vi "211104-VNA RP FLAT.vi"() -> ()   [LabVIEW 2021]
uses:
  b7fd31b3-4c8f-4ae8-a038-7c142e2eb182.vi
  <vilib>/Analysis/baseanly.llb/Mean (DBL).vi
  <vilib>/Utility/file.llb/Write Delimited Spreadsheet (DBL).vi
  <vilib>/Comparison/Equal/Equal Functor/Equal Functor.lvclass
  <vilib>/Analysis/NI_AALBase.lvlib
panel:
  in  "RP VNA SETTING":T1={"F start"=200000, "F stop"=2000500, "Sweep size"=1000, "Decimation"=5000, "F_corr"=0, "Ph_OUT1"=0, "Ph_OUT2"=0, "OUT_Lvl1"=32700, "OUT_Lvl2"=32700, "GPIO"=0}
  in  "Amplitude(1V)":dbl=0.3 format="%#_13g"
  out "RP CONNECT":bool
  in  "VOA Calibration cluster":cluster{"PUMP":dbl[], "PROBE":dbl[]}
  out "TRACK DATA REL NO SMOOTHING":dbl[][](array[numeric])
  out "TRACK DATA ABS NO SMOOTHING":dbl[][](array[numeric])
  in  "BTN SAVE TRACK":bool
  in  "BTN STOP TRACK":bool
  out "TRACK REPOSITERY":path
  out "TRACK DATA REL":dbl[][](array[numeric])
  out "TRACK DATA ABS":dbl[][](array[numeric])
  out "Track File List":path[](array[path])
  out "Track Repositery List":path[](array[path])
  out "CHANNEL CHOSEN":i32
  in  "TRACK-STOP":bool
  out "STATUS":string="STOP"
  out "track data":dbl[](array[numeric])=[495490.5081042979, 495481.56129759253, 495478.2328599854, 495479.84884744807, 495476.377462383, 495478.7819904735]
  out "Information tips":string
  in  "PANEL VNA":bool
  in  "PANEL TRACKING":bool
  in  "BTN STOP":bool
  in  "PANEL GENERAL SETTINGS":bool
  in  "PANEL TRACK SETTINGS":bool
  out "MAIN TAB":T2(tab)
  out "ACQ Indicator":bool
  in  "PUMP":dbl(slide)=100.0 min=0.0 max=100.0 step=0.1 scale=0.0..100.0
  in  "PROBE":dbl(slide)=100.0 min=0.0 max=100.0 step=0.1 scale=0.0..100.0
  in  "BTN RESET VNA":bool
  in  "SPAN":dbl=1900.0 format="%#5.1f"
  in  "STOP":dbl=2000.0 format="%#5.1f"
  in  "CENTER":dbl=1050.0 format="%#5.1f"
  in  "BTN SAVE VNA STG TO TRACK":bool
  in  "BTN AF VNA":bool
  out "MAGNITUDE/PHASE":cluster{cluster{dbl, dbl}[]}[](graph)
  in  "CHANNEL CHOICE VNA":T3(radio)
  in  "BTN Center to max":bool
  in  "BTN ZOOM-":bool
  in  "BTN ZOOM+":bool
  in  "START":dbl=200.0 format="%#5.1f"
  out "SPACING":dbl=1900.0 min=0.0 max=100.0 step=0.5 format="%#5.1f"
  in  "Points N°":i32=1000 min=600 max=5000 step=1 format="%#4.4g"
  in  "BTN LOOP VNA":bool
  in  "BTN RUN VNA":bool
  in  "Hide/Show track data channel":bool[](array[boolean])
  in  "BTN AUTOSAVE RAW DATA":bool=TRUE
  in  "COMMENTS":string
  in  "ASSAY NAME":string
  in  "DELAY AFTER SWITCH (s)":i32
  in  "N°POINTS TO DISPLAY":i32=200
  in  "DISPLAY OPTION":u16(ring) items=["Absolute frequency", "Relative frequency (ppm)"]
  in  "DELAY BETWEEN TRIG (s)":i32
  in  "AVERAGE/POINT":dbl=1.0
  out "LIVE TRACK":dbl[][](graph)
  out "CHANNELS IND TRACK":T3(radio)
  in  "BTN RUN TRACK":bool
  in  "TEMPORAL SMOOTHING":i32=15
  in  "BTN NEW TRACK":bool
  in  "BTN PAUSE TRACK":bool
  in  "CHANNELS PARAMETERS":T4(array[cluster])=[{"START 2"=200.0, "STOP 2"=2000.5, "CENTER 2"=1050.0, "SPAN 2"=1800.0, "CHANNEL TRACK ?"=FALSE, "PUMP"=100.0, "PROBE"=100.0, "Points N° 2"=1000, "SPACING 2"=100.0}, {"START 2"=200.0, "STOP 2"=2000.0, "CENTER 2"=1100.0, "SPAN 2"=1800.0, "CHANNEL TRACK ?"=FALSE, "PUMP"=100.0, "PROBE"=100.0, "Points N° 2"=1000, "SPACING 2"=1800.0}, {"START 2"=200.0, "STOP 2"=2000.0, "CENTER 2"=1100.0, "SPAN 2"=1800.0, "CHANNEL TRACK ?"=FALSE, "PUMP"=100.0, "PROBE"=100.0, "Points N° 2"=1000, "SPACING 2"=1800.0}, {"START 2"=200.0, "STOP 2"=2000.0, "CENTER 2"=1100.0, "SPAN 2"=1800.0, "CHANNEL TRACK ?"=FALSE, "PUMP"=100.0, "PROBE"=100.0, "Points N° 2"=1000, "SPACING 2"=1800.0}, {"START 2"=200.0, "STOP 2"=2000.0, "CENTER 2"=1100.0, "SPAN 2"=1800.0, "CHANNEL TRACK ?"=FALSE, "PUMP"=100.0, "PROBE"=100.0, "Points N° 2"=1000, "SPACING 2"=1800.0}, {"START 2"=200.0, "STOP 2"=2000.0, "CENTER 2"=1100.0, "SPAN 2"=1800.0, "CHANNEL TRACK ?"=FALSE, "PUMP"=100.0, "PROBE"=100.0, "Points N° 2"=1000, "SPACING 2"=1800.0}, {"START 2"=200.0, "STOP 2"=2000.0, "CENTER 2"=1100.0, "SPAN 2"=1800.0, "CHANNEL TRACK ?"=FALSE, "PUMP"=100.0, "PROBE"=100.0, "Points N° 2"=1000, "SPACING 2"=1800.0}, {"START 2"=200.0, "STOP 2"=2000.0, "CENTER 2"=1100.0, "SPAN 2"=1800.0, "CHANNEL TRACK ?"=FALSE, "PUMP"=100.0, "PROBE"=100.0, "Points N° 2"=1000, "SPACING 2"=1800.0}, {"START 2"=200.0, "STOP 2"=2000.0, "CENTER 2"=1100.0, "SPAN 2"=1800.0, "CHANNEL TRACK ?"=FALSE, "PUMP"=100.0, "PROBE"=100.0, "Points N° 2"=1000, "SPACING 2"=1800.0}, {"START 2"=200.0, "STOP 2"=2000.0, "CENTER 2"=1100.0, "SPAN 2"=1800.0, "CHANNEL TRACK ?"=FALSE, "PUMP"=100.0, "PROBE"=100.0, "Points N° 2"=1000, "SPACING 2"=1800.0}, {"START 2"=200.0, "STOP 2"=2000.0, "CENTER 2"=1100.0, "SPAN 2"=1800.0, "CHANNEL TRACK ?"=FALSE, "PUMP"=100.0, "PROBE"=100.0, "Points N° 2"=1000, "SPACING 2"=1800.0}, {"START 2"=200.0, "STOP 2"=2000.0, "CENTER 2"=1100.0, "SPAN 2"=1800.0, "CHANNEL TRACK ?"=FALSE, "PUMP"=100.0, "PROBE"=100.0, "Points N° 2"=1000, "SPACING 2"=1800.0}, {"START 2"=200.0, "STOP 2"=2000.0, "CENTER 2"=1100.0, "SPAN 2"=1800.0, "CHANNEL TRACK ?"=FALSE, "PUMP"=100.0, "PROBE"=100.0, "Points N° 2"=1000, "SPACING 2"=1800.0}, {"START 2"=200.0, "STOP 2"=2000.0, "CENTER 2"=1100.0, "SPAN 2"=1800.0, "CHANNEL TRACK ?"=FALSE, "PUMP"=100.0, "PROBE"=100.0, "Points N° 2"=1000, "SPACING 2"=1800.0}, {"START 2"=200.0, "STOP 2"=2000.0, "CENTER 2"=1100.0, "SPAN 2"=1800.0, "CHANNEL TRACK ?"=FALSE, "PUMP"=100.0, "PROBE"=100.0, "Points N° 2"=1000, "SPACING 2"=1800.0}, {"START 2"=200.0, "STOP 2"=2000.0, "CENTER 2"=1100.0, "SPAN 2"=1800.0, "CHANNEL TRACK ?"=FALSE, "PUMP"=100.0, "PROBE"=100.0, "Points N° 2"=1000, "SPACING 2"=1800.0}] {"SPACING 2" min=0.0 max=100.0 step=0.5; "Points N° 2" min=0 max=100 step=1; "PROBE" min=0.0 max=100.0 step=0.5; "PUMP" min=0.0 max=100.0 step=0.5}
  out "CHANNEL IND SETTINGS":T5(radio)
  in  "TRACK DATA PARAMETERS":cluster{"MAIN FOLDER":path}={"MAIN FOLDER"=path "C:/SensWay Data"}
  in  "SPECTRUM POST PROCESSING PARAMETERS":cluster{"N° SMOOTHING POINTS":i32}={"N° SMOOTHING POINTS"=50}
  in  "AUTOFOCUS PARAMETERS":cluster{"ITERATIONS":i32}={"ITERATIONS"=5}
  in  "CHANNELS":T6
  in  "NETWORK PARAMETERS":cluster{"RP-IP 1":string, "RP-IP 2":string}={"RP-IP 1"="192.168.0.3", "RP-IP 2"="192.168.0.4"}
  in  "VNA DATA CLUSTER":T7
  in  "TRACK DATA CLUSTER":cluster{"CHANNEL":dbl, "KPI 1 TRACK":ext[]}
  out "LOOP ACT":bool
  out "RAW Freq table":dbl[](array[numeric])=[200000.0, 201802.3023023023, 203604.6046046046, 205406.9069069069, 207209.20920920922, 209011.51151151152, 210813.81381381382, 212616.1161161161, 214418.4184184184, 216220.7207207207, 218023.02302302304, 219825.32532532534, 221627.62762762763, 223429.92992992993, 225232.23223223223, 227034.53453453453, 228836.83683683682, 230639.13913913915, 232441.44144144145, 234243.74374374375, 236046.04604604605, 237848.34834834834, 239650.65065065064, 241452.95295295294, 243255.25525525527, 245057.55755755756, 246859.85985985986, 248662.16216216216, 250464.46446446446, 252266.76676676676, 254069.06906906905, 255871.37137137138, 257673.67367367368, 259475.97597597598, 261278.27827827827, 263080.5805805806, 264882.8828828829, 266685.18518518517, 268487.4874874875, 270289.7897897898, 272092.0920920921, 273894.39439439436, 275696.6966966967, 277498.998998999, 279301.3013013013, 281103.6036036036, 282905.9059059059, 284708.2082082082, 286510.51051051053, 288312.8128128128, 290115.1151151151, 291917.4174174174, 293719.7197197197, 295522.02202202205, 297324.3243243243, 299126.6266266266, 300928.9289289289, 302731.23123123124, 304533.5335335335, 306335.83583583584, 308138.1381381381, 309940.44044044043, 311742.74274274276, 313545.04504504503, 315347.34734734736, 317149.6496496496, 318951.95195195195, 320754.2542542543, 322556.55655655655, 324358.8588588588, 326161.16116116114, 327963.4634634635, 329765.76576576574, 331568.06806806807, 333370.37037037034, 335172.67267267266, 336974.974974975, 338777.27727727726, 340579.5795795796, 342381.88188188185, 344184.1841841842, 345986.4864864865, 347788.7887887888, 349591.09109109105, 351393.3933933934, 353195.6956956957, 354997.997997998, 356800.3003003003, 358602.60260260256, 360404.9049049049, 362207.2072072072, 364009.50950950955, 365811.8118118118, 367614.1141141141, 369416.4164164164, 371218.71871871874, 373021.021021021, 374823.3233233233, 376625.6256256256, 378427.9279279279, 380230.23023023026, 382032.5325325325, 383834.8348348348, 385637.1371371371, 387439.43943943945, 389241.7417417418, 391044.04404404404, 392846.3463463463, 394648.64864864864, 396450.95095095097, 398253.25325325324, 400055.5555555555, 401857.85785785783, 403660.16016016016, 405462.4624624625, 407264.76476476475, 409067.067067067, 410869.36936936935, 412671.6716716717, 414473.973973974, 416276.2762762763, 418078.57857857854, 419880.88088088087, 421683.1831831832, 423485.48548548546, 425287.7877877878, 427090.09009009006, 428892.3923923924, 430694.6946946947, 432496.996996997, 434299.29929929925, 436101.6016016016, 437903.9039039039, 439706.20620620623, 441508.5085085085, 443310.81081081077, 445113.1131131131, 446915.4154154154, 448717.7177177177, 450520.02002002, 452322.3223223223, 454124.6246246246, 455926.92692692694, 457729.2292292292, 459531.5315315315, 461333.8338338338, 463136.13613613613, 464938.4384384384, 466740.74074074073, 468543.04304304306, 470345.3453453453, 472147.64764764765, 473949.9499499499, 475752.25225225225, 477554.5545545545, 479356.85685685684, 481159.1591591592, 482961.46146146144, 484763.76376376377, 486566.06606606604, 488368.36836836836, 490170.67067067063, 491972.97297297296, 493775.2752752753, 495577.57757757755, 497379.8798798799, 499182.18218218215, 500984.4844844845, 502786.78678678675, 504589.0890890891, 506391.3913913914, 508193.69369369367, 509995.995995996, 511798.29829829826, 513600.6006006006, 515402.90290290286, 517205.2052052052, 519007.5075075075, 520809.8098098098, 522612.1121121121, 524414.4144144144, 526216.7167167168, 528019.0190190191, 529821.3213213213, 531623.6236236236, 533425.9259259258, 535228.2282282282, 537030.5305305305, 538832.8328328328, 540635.1351351351, 542437.4374374375, 544239.7397397398, 546042.042042042, 547844.3443443443, 549646.6466466465, 551448.9489489489, 553251.2512512512, 555053.5535535535, 556855.8558558559, 558658.1581581582, 560460.4604604605, 562262.7627627627, 564065.065065065, 565867.3673673674, 567669.6696696696, 569471.9719719719, 571274.2742742742, 573076.5765765766, 574878.8788788789, 576681.1811811812, 578483.4834834835, 580285.7857857858, 582088.0880880881, 583890.3903903903, 585692.6926926926, 587494.994994995, 589297.2972972973, 591099.5995995996, 592901.9019019019, 594704.2042042043, 596506.5065065065, 598308.8088088088, 600111.111111111, 601913.4134134133, 603715.7157157157, 605518.018018018, 607320.3203203203, 609122.6226226226, 610924.924924925, 612727.2272272272, 614529.5295295295, 616331.8318318318, 618134.134134134, 619936.4364364364, 621738.7387387387, 623541.041041041, 625343.3433433434, 627145.6456456457, 628947.947947948, 630750.2502502502, 632552.5525525525, 634354.8548548548, 636157.1571571571, 637959.4594594594, 639761.7617617617, 641564.0640640641, 643366.3663663664, 645168.6686686687, 646970.9709709709, 648773.2732732733, 650575.5755755756, 652377.8778778778, 654180.1801801801, 655982.4824824824, 657784.7847847848, 659587.0870870871, 661389.3893893894, 663191.6916916918, 664993.993993994, 666796.2962962963, 668598.5985985985, 670400.9009009008, 672203.2032032032, 674005.5055055055, 675807.8078078078, 677610.1101101101, 679412.4124124125, 681214.7147147147, 683017.017017017, 684819.3193193192, 686621.6216216215, 688423.9239239239, 690226.2262262262, 692028.5285285285, 693830.8308308308, 695633.1331331332, 697435.4354354354, 699237.7377377377, 701040.04004004, 702842.3423423423, 704644.6446446446, 706446.9469469469, 708249.2492492492, 710051.5515515516, 711853.8538538539, 713656.1561561562, 715458.4584584584, 717260.7607607607, 719063.063063063, 720865.3653653653, 722667.6676676676, 724469.9699699699, 726272.2722722723, 728074.5745745746, 729876.8768768768, 731679.1791791791, 733481.4814814815, 735283.7837837838, 737086.0860860861, 738888.3883883883, 740690.6906906907, 742492.992992993, 744295.2952952953, 746097.5975975975, 747899.8998998998, 749702.2022022022, 751504.5045045045, 753306.8068068068, 755109.109109109, 756911.4114114114, 758713.7137137137, 760516.016016016, 762318.3183183183, 764120.6206206206, 765922.9229229229, 767725.2252252252, 769527.5275275275, 771329.8298298299, 773132.1321321321, 774934.4344344344, 776736.7367367367, 778539.039039039, 780341.3413413413, 782143.6436436436, 783945.9459459459, 785748.2482482482, 787550.5505505506, 789352.8528528528, 791155.1551551551, 792957.4574574574, 794759.7597597598, 796562.0620620621, 798364.3643643643, 800166.6666666666, 801968.968968969, 803771.2712712713, 805573.5735735735, 807375.8758758758, 809178.1781781781, 810980.4804804805, 812782.7827827828, 814585.085085085, 816387.3873873873, 818189.6896896897, 819991.991991992, 821794.2942942943, 823596.5965965965, 825398.8988988989, 827201.2012012012, 829003.5035035035, 830805.8058058057, 832608.108108108, 834410.4104104104, 836212.7127127127, 838015.015015015, 839817.3173173172, 841619.6196196196, 843421.9219219219, 845224.2242242242, 847026.5265265265, 848828.8288288288, 850631.1311311311, 852433.4334334334, 854235.7357357357, 856038.0380380381, 857840.3403403403, 859642.6426426426, 861444.9449449449, 863247.2472472473, 865049.5495495495, 866851.8518518518, 868654.1541541541, 870456.4564564564, 872258.7587587588, 874061.061061061, 875863.3633633633, 877665.6656656656, 879467.967967968, 881270.2702702703, 883072.5725725725, 884874.8748748748, 886677.1771771772, 888479.4794794795, 890281.7817817817, 892084.084084084, 893886.3863863864, 895688.6886886887, 897490.990990991, 899293.2932932932, 901095.5955955955, 902897.8978978979, 904700.2002002002, 906502.5025025025, 908304.8048048047, 910107.1071071071, 911909.4094094094, 913711.7117117117, 915514.0140140139, 917316.3163163163, 919118.6186186186, 920920.9209209209, 922723.2232232232, 924525.5255255254, 926327.8278278278, 928130.1301301301, 929932.4324324324, 931734.7347347348, 933537.037037037, 935339.3393393393, 937141.6416416416, 938943.943943944, 940746.2462462463, 942548.5485485485, 944350.8508508508, 946153.1531531531, 947955.4554554555, 949757.7577577577, 951560.06006006, 953362.3623623623, 955164.6646646647, 956966.966966967, 958769.2692692692, 960571.5715715715, 962373.8738738738, 964176.1761761762, 965978.4784784785, 967780.7807807807, 969583.083083083, 971385.3853853854, 973187.6876876877, 974989.9899899899, 976792.2922922922, 978594.5945945946, 980396.8968968969, 982199.1991991992, 984001.5015015014, 985803.8038038037, 987606.1061061061, 989408.4084084084, 991210.7107107107, 993013.0130130129, 994815.3153153153, 996617.6176176176, 998419.9199199199, 1000222.2222222221, 1002024.5245245245, 1003826.8268268268, 1005629.1291291291, 1007431.4314314314, 1009233.7337337337, 1011036.036036036, 1012838.3383383383, 1014640.6406406406, 1016442.942942943, 1018245.2452452452, 1020047.5475475475, 1021849.8498498498, 1023652.1521521521, 1025454.4544544544, 1027256.7567567567, 1029059.059059059, 1030861.3613613613, 1032663.6636636637, 1034465.9659659659, 1036268.2682682682, 1038070.5705705705, 1039872.8728728729, 1041675.1751751752, 1043477.4774774774, 1045279.7797797797, 1047082.082082082, 1048884.3843843844, 1050686.6866866867, 1052488.988988989, 1054291.2912912914, 1056093.5935935937, 1057895.895895896, 1059698.198198198, 1061500.5005005004, 1063302.8028028028, 1065105.105105105, 1066907.4074074074, 1068709.7097097095, 1070512.0120120118, 1072314.3143143142, 1074116.6166166165, 1075918.9189189188, 1077721.2212212211, 1079523.5235235235, 1081325.8258258258, 1083128.1281281281, 1084930.4304304305, 1086732.7327327328, 1088535.035035035, 1090337.3373373374, 1092139.6396396398, 1093941.9419419419, 1095744.2442442442, 1097546.5465465465, 1099348.8488488488, 1101151.1511511512, 1102953.4534534533, 1104755.7557557556, 1106558.058058058, 1108360.3603603602, 1110162.6626626626, 1111964.964964965, 1113767.2672672672, 1115569.5695695695, 1117371.8718718719, 1119174.1741741742, 1120976.4764764765, 1122778.7787787789, 1124581.0810810812, 1126383.3833833835, 1128185.6856856856, 1129987.987987988, 1131790.2902902903, 1133592.5925925926, 1135394.894894895, 1137197.197197197, 1138999.4994994993, 1140801.8018018017, 1142604.104104104, 1144406.4064064063, 1146208.7087087086, 1148011.011011011, 1149813.3133133133, 1151615.6156156156, 1153417.917917918, 1155220.2202202203, 1157022.5225225226, 1158824.824824825, 1160627.1271271273, 1162429.4294294294, 1164231.7317317317, 1166034.034034034, 1167836.3363363363, 1169638.6386386384, 1171440.9409409408, 1173243.243243243, 1175045.5455455454, 1176847.8478478477, 1178650.15015015, 1180452.4524524524, 1182254.7547547547, 1184057.057057057, 1185859.3593593594, 1187661.6616616617, 1189463.963963964, 1191266.2662662663, 1193068.5685685687, 1194870.8708708708, 1196673.173173173, 1198475.4754754754, 1200277.7777777778, 1202080.08008008, 1203882.3823823822, 1205684.6846846845, 1207486.9869869868, 1209289.2892892892, 1211091.5915915915, 1212893.8938938938, 1214696.1961961961, 1216498.4984984985, 1218300.8008008008, 1220103.103103103, 1221905.4054054054, 1223707.7077077078, 1225510.01001001, 1227312.3123123124, 1229114.6146146145, 1230916.9169169168, 1232719.2192192192, 1234521.5215215215, 1236323.8238238238, 1238126.126126126, 1239928.4284284282, 1241730.7307307306, 1243533.033033033, 1245335.3353353352, 1247137.6376376376, 1248939.9399399399, 1250742.2422422422, 1252544.5445445445, 1254346.8468468469, 1256149.1491491492, 1257951.4514514515, 1259753.7537537536, 1261556.056056056, 1263358.3583583583, 1265160.6606606606, 1266962.962962963, 1268765.2652652652, 1270567.5675675676, 1272369.86986987, 1274172.1721721722, 1275974.4744744743, 1277776.7767767766, 1279579.079079079, 1281381.3813813813, 1283183.6836836836, 1284985.985985986, 1286788.2882882883, 1288590.5905905906, 1290392.892892893, 1292195.195195195, 1293997.4974974974, 1295799.7997997997, 1297602.102102102, 1299404.4044044043, 1301206.7067067067, 1303009.009009009, 1304811.3113113113, 1306613.6136136136, 1308415.915915916, 1310218.218218218, 1312020.5205205204, 1313822.8228228227, 1315625.125125125, 1317427.4274274274, 1319229.7297297297, 1321032.032032032, 1322834.3343343344, 1324636.6366366367, 1326438.9389389388, 1328241.241241241, 1330043.5435435434, 1331845.8458458458, 1333648.148148148, 1335450.4504504504, 1337252.7527527527, 1339055.055055055, 1340857.3573573574, 1342659.6596596597, 1344461.9619619618, 1346264.2642642641, 1348066.5665665665, 1349868.8688688688, 1351671.1711711711, 1353473.4734734735, 1355275.7757757758, 1357078.078078078, 1358880.3803803804, 1360682.6826826825, 1362484.9849849849, 1364287.2872872872, 1366089.5895895895, 1367891.8918918918, 1369694.1941941942, 1371496.4964964965, 1373298.7987987988, 1375101.1011011011, 1376903.4034034032, 1378705.7057057056, 1380508.008008008, 1382310.3103103102, 1384112.6126126125, 1385914.9149149149, 1387717.2172172172, 1389519.5195195195, 1391321.8218218219, 1393124.1241241242, 1394926.4264264263, 1396728.7287287286, 1398531.031031031, 1400333.3333333333, 1402135.6356356356, 1403937.937937938, 1405740.2402402402, 1407542.5425425426, 1409344.844844845, 1411147.147147147, 1412949.4494494493, 1414751.7517517516, 1416554.054054054, 1418356.3563563563, 1420158.6586586586, 1421960.960960961, 1423763.2632632633, 1425565.5655655656, 1427367.867867868, 1429170.17017017, 1430972.4724724723, 1432774.7747747747, 1434577.077077077, 1436379.3793793793, 1438181.6816816817, 1439983.983983984, 1441786.2862862863, 1443588.5885885886, 1445390.8908908907, 1447193.193193193, 1448995.4954954954, 1450797.7977977977, 1452600.1001001, 1454402.4024024024, 1456204.7047047047, 1458007.007007007, 1459809.3093093093, 1461611.6116116114, 1463413.9139139138, 1465216.216216216, 1467018.5185185184, 1468820.8208208208, 1470623.123123123, 1472425.4254254254, 1474227.7277277277, 1476030.03003003, 1477832.3323323324, 1479634.6346346345, 1481436.9369369368, 1483239.2392392391, 1485041.5415415415, 1486843.8438438438, 1488646.146146146, 1490448.4484484484, 1492250.7507507508, 1494053.053053053, 1495855.3553553552, 1497657.6576576575, 1499459.9599599598, 1501262.2622622622, 1503064.5645645645, 1504866.8668668668, 1506669.1691691692, 1508471.4714714715, 1510273.7737737738, 1512076.0760760761, 1513878.3783783782, 1515680.6806806806, 1517482.9829829829, 1519285.2852852852, 1521087.5875875875, 1522889.8898898899, 1524692.1921921922, 1526494.4944944945, 1528296.7967967968, 1530099.099099099, 1531901.4014014013, 1533703.7037037036, 1535506.006006006, 1537308.3083083082, 1539110.6106106106, 1540912.912912913, 1542715.2152152152, 1544517.5175175176, 1546319.8198198196, 1548122.122122122, 1549924.4244244243, 1551726.7267267266, 1553529.029029029, 1555331.3313313313, 1557133.6336336336, 1558935.935935936, 1560738.2382382383, 1562540.5405405406, 1564342.8428428427, 1566145.145145145, 1567947.4474474473, 1569749.7497497497, 1571552.052052052, 1573354.3543543543, 1575156.6566566566, 1576958.958958959, 1578761.2612612613, 1580563.5635635634, 1582365.8658658657, 1584168.168168168, 1585970.4704704704, 1587772.7727727727, 1589575.075075075, 1591377.3773773774, 1593179.6796796797, 1594981.981981982, 1596784.2842842843, 1598586.5865865864, 1600388.8888888888, 1602191.191191191, 1603993.4934934934, 1605795.7957957957, 1607598.098098098, 1609400.4004004004, 1611202.7027027027, 1613005.005005005, 1614807.3073073071, 1616609.6096096095, 1618411.9119119118, 1620214.2142142141, 1622016.5165165165, 1623818.8188188188, 1625621.121121121, 1627423.4234234234, 1629225.7257257258, 1631028.0280280279, 1632830.3303303302, 1634632.6326326325, 1636434.9349349348, 1638237.2372372372, 1640039.5395395395, 1641841.8418418418, 1643644.1441441441, 1645446.4464464465, 1647248.7487487488, 1649051.051051051, 1650853.3533533532, 1652655.6556556555, 1654457.9579579579, 1656260.2602602602, 1658062.5625625625, 1659864.8648648649, 1661667.1671671672, 1663469.4694694695, 1665271.7717717716, 1667074.074074074, 1668876.3763763763, 1670678.6786786786, 1672480.980980981, 1674283.2832832832, 1676085.5855855856, 1677887.887887888, 1679690.1901901902, 1681492.4924924925, 1683294.7947947946, 1685097.097097097, 1686899.3993993993, 1688701.7017017016, 1690504.004004004, 1692306.3063063063, 1694108.6086086086, 1695910.910910911, 1697713.2132132133, 1699515.5155155153, 1701317.8178178177, 1703120.12012012, 1704922.4224224223, 1706724.7247247247, 1708527.027027027, 1710329.3293293293, 1712131.6316316316, 1713933.933933934, 1715736.236236236, 1717538.5385385384, 1719340.8408408407, 1721143.143143143, 1722945.4454454454, 1724747.7477477477, 1726550.05005005, 1728352.3523523523, 1730154.6546546547, 1731956.956956957, 1733759.259259259, 1735561.5615615614, 1737363.8638638637, 1739166.166166166, 1740968.4684684684, 1742770.7707707707, 1744573.073073073, 1746375.3753753754, 1748177.6776776777, 1749979.9799799798, 1751782.2822822821, 1753584.5845845845, 1755386.8868868868, 1757189.189189189, 1758991.4914914914, 1760793.7937937938, 1762596.096096096, 1764398.3983983984, 1766200.7007007005, 1768003.0030030028, 1769805.3053053052, 1771607.6076076075, 1773409.9099099098, 1775212.2122122122, 1777014.5145145145, 1778816.8168168168, 1780619.1191191191, 1782421.4214214215, 1784223.7237237236, 1786026.0260260259, 1787828.3283283282, 1789630.6306306305, 1791432.9329329329, 1793235.2352352352, 1795037.5375375375, 1796839.8398398398, 1798642.1421421422, 1800444.4444444443, 1802246.7467467466, 1804049.049049049, 1805851.3513513512, 1807653.6536536536, 1809455.955955956, 1811258.2582582582, 1813060.5605605606, 1814862.8628628629, 1816665.1651651652, 1818467.4674674673, 1820269.7697697696, 1822072.072072072, 1823874.3743743743, 1825676.6766766766, 1827478.978978979, 1829281.2812812813, 1831083.5835835836, 1832885.885885886, 1834688.188188188, 1836490.4904904903, 1838292.7927927927, 1840095.095095095, 1841897.3973973973, 1843699.6996996996, 1845502.002002002, 1847304.3043043043, 1849106.6066066066, 1850908.9089089087, 1852711.211211211, 1854513.5135135134, 1856315.8158158157, 1858118.118118118, 1859920.4204204204, 1861722.7227227227, 1863525.025025025, 1865327.3273273273, 1867129.6296296297, 1868931.9319319318, 1870734.234234234, 1872536.5365365364, 1874338.8388388387, 1876141.141141141, 1877943.4434434434, 1879745.7457457457, 1881548.048048048, 1883350.3503503504, 1885152.6526526525, 1886954.9549549548, 1888757.2572572571, 1890559.5595595594, 1892361.8618618618, 1894164.164164164, 1895966.4664664664, 1897768.7687687688, 1899571.071071071, 1901373.3733733734, 1903175.6756756755, 1904977.9779779778, 1906780.2802802802, 1908582.5825825825, 1910384.8848848848, 1912187.1871871871, 1913989.4894894895, 1915791.7917917918, 1917594.0940940941, 1919396.3963963962, 1921198.6986986985, 1923001.0010010009, 1924803.3033033032, 1926605.6056056055, 1928407.9079079079, 1930210.2102102102, 1932012.5125125125, 1933814.8148148148, 1935617.117117117, 1937419.4194194193, 1939221.7217217216, 1941024.024024024, 1942826.3263263262, 1944628.6286286286, 1946430.930930931, 1948233.2332332332, 1950035.5355355355, 1951837.8378378379, 1953640.14014014, 1955442.4424424423, 1957244.7447447446, 1959047.047047047, 1960849.3493493493, 1962651.6516516516, 1964453.953953954, 1966256.2562562563, 1968058.5585585586, 1969860.8608608607, 1971663.163163163, 1973465.4654654653, 1975267.7677677677, 1977070.07007007, 1978872.3723723723, 1980674.6746746746, 1982476.976976977, 1984279.2792792793, 1986081.5815815816, 1987883.8838838837, 1989686.186186186, 1991488.4884884884, 1993290.7907907907, 1995093.093093093, 1996895.3953953953, 1998697.6976976977, 2000500.0]
  in  "ENABLE INTERNAL MODULATION":bool=TRUE
  in  "VNA DATA CLUSTER TBL":T8(array[cluster])=[{"CHANNEL"=0.0, "FREQUENCY TABLE"=[0.0], "MAGNITUDE TABLE"=[0.0], "PHASE TABLE"=[0.0]}, {"CHANNEL"=1.0, "FREQUENCY TABLE"=[], "MAGNITUDE TABLE"=[], "PHASE TABLE"=[]}, {"CHANNEL"=2.0, "FREQUENCY TABLE"=[], "MAGNITUDE TABLE"=[], "PHASE TABLE"=[]}, {"CHANNEL"=3.0, "FREQUENCY TABLE"=[], "MAGNITUDE TABLE"=[], "PHASE TABLE"=[]}, {"CHANNEL"=4.0, "FREQUENCY TABLE"=[], "MAGNITUDE TABLE"=[], "PHASE TABLE"=[]}, {"CHANNEL"=5.0, "FREQUENCY TABLE"=[], "MAGNITUDE TABLE"=[], "PHASE TABLE"=[]}, {"CHANNEL"=6.0, "FREQUENCY TABLE"=[], "MAGNITUDE TABLE"=[], "PHASE TABLE"=[]}, {"CHANNEL"=7.0, "FREQUENCY TABLE"=[], "MAGNITUDE TABLE"=[], "PHASE TABLE"=[]}, {"CHANNEL"=8.0, "FREQUENCY TABLE"=[], "MAGNITUDE TABLE"=[], "PHASE TABLE"=[]}, {"CHANNEL"=9.0, "FREQUENCY TABLE"=[], "MAGNITUDE TABLE"=[], "PHASE TABLE"=[]}, {"CHANNEL"=10.0, "FREQUENCY TABLE"=[], "MAGNITUDE TABLE"=[], "PHASE TABLE"=[]}, {"CHANNEL"=11.0, "FREQUENCY TABLE"=[], "MAGNITUDE TABLE"=[], "PHASE TABLE"=[]}, {"CHANNEL"=12.0, "FREQUENCY TABLE"=[], "MAGNITUDE TABLE"=[], "PHASE TABLE"=[]}, {"CHANNEL"=13.0, "FREQUENCY TABLE"=[], "MAGNITUDE TABLE"=[], "PHASE TABLE"=[]}, {"CHANNEL"=14.0, "FREQUENCY TABLE"=[], "MAGNITUDE TABLE"=[], "PHASE TABLE"=[]}, {"CHANNEL"=15.0, "FREQUENCY TABLE"=[], "MAGNITUDE TABLE"=[], "PHASE TABLE"=[]}]
  in  "TRACK DATA CLUSTER TBL":cluster{"CHANNEL":dbl, "KPI 1 TRACK":ext[]}[](array[cluster])
  in  "VNA Settings cluster":T9={"START 2"=200.0, "STOP 2"=2000.5, "CENTER 2"=1050.0, "SPAN 2"=1901.0, "CHANNEL TRACK ?"=FALSE, "PUMP"=100.0, "PROBE"=100.0, "Points N° 2"=1000, "SPACING 2"=1901.0} {"SPACING 2" min=0.0 max=100.0 step=0.5; "Points N° 2" min=0 max=100 step=1; "PROBE" min=0.0 max=100.0 step=0.5; "PUMP" min=0.0 max=100.0 step=0.5}
  # "E"
  # "POINTS"
  # "SPACING"
  # "TRACK ?"
  # "START"
  # "STOP"
  # "CENTER"
  # "SPAN"
  # "PROBE"
  # "PUMP"
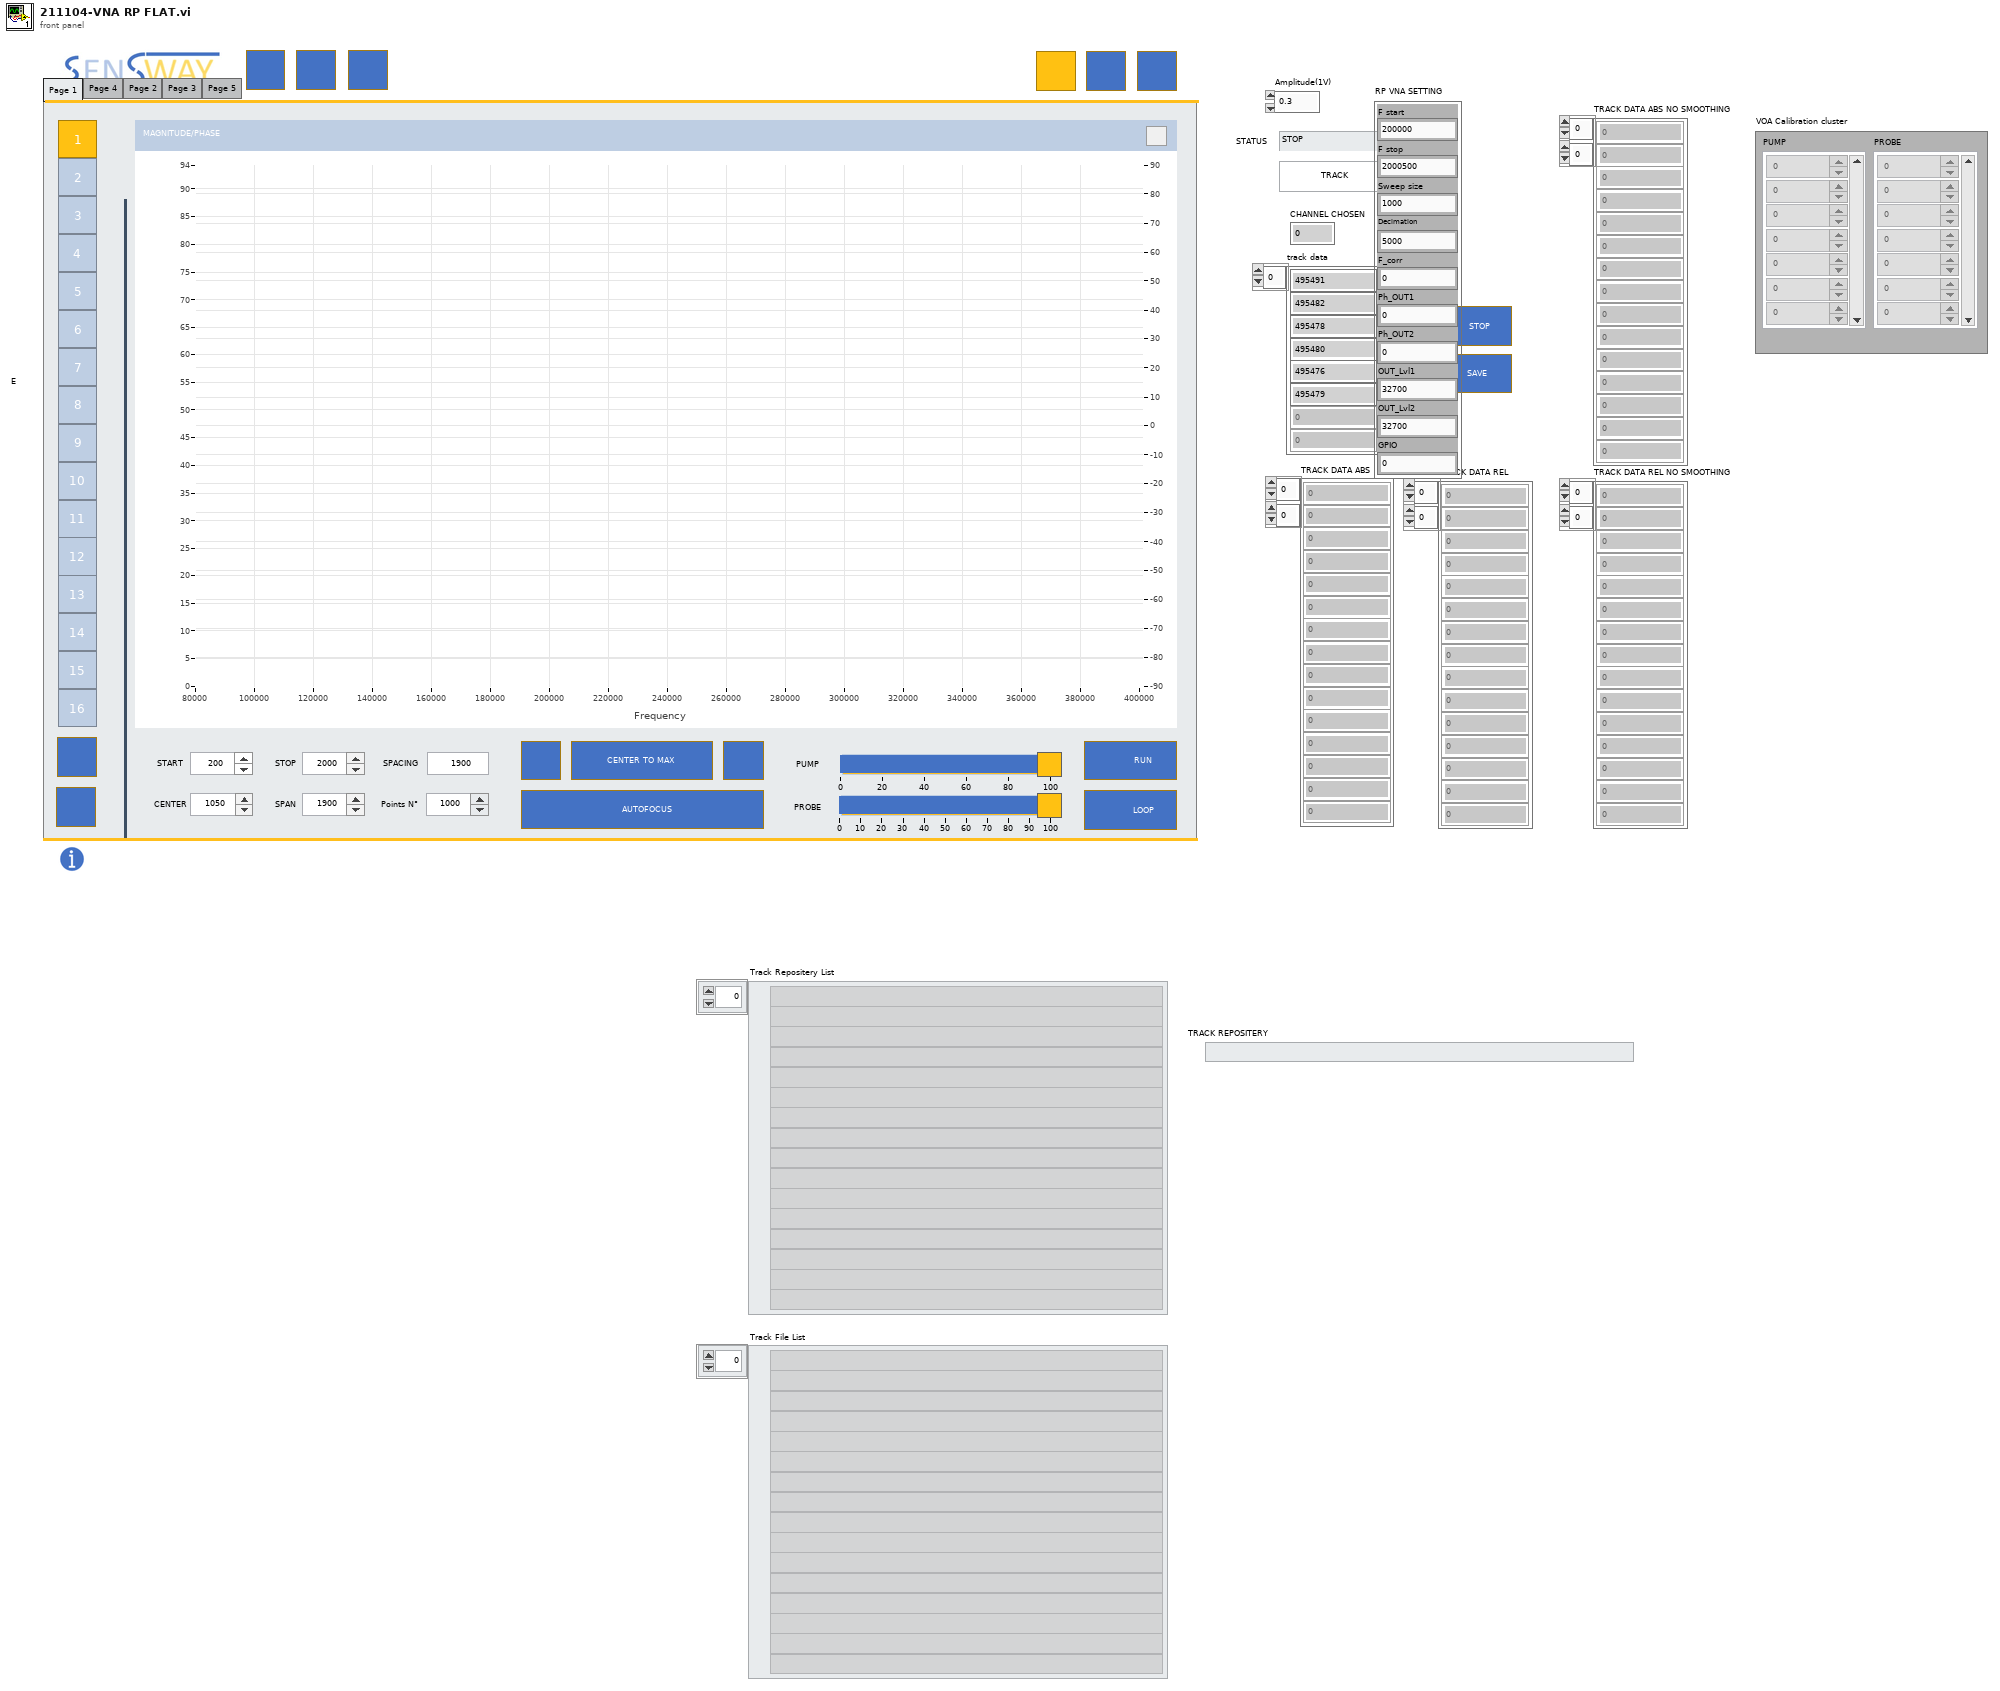
[diagram p1: front panel]
types:
  T1 = cluster{"F start":u32, "F stop":u32, "Sweep size":u32, "Decimation":u32, "F_corr":u32, "Ph_OUT1":u32, "Ph_OUT2":u32, "OUT_Lvl1":u32, "OUT_Lvl2":u32, "GPIO":u32}
  T2 = enum32{"Page 1", "Page 4", "Page 2", "Page 3", "Page 5"}
  T3 = enum32{"Button 1", "Button 2", "Button 3", "Sélection radio 4", "Sélection radio 5", "Sélection radio 6", "Sélection radio 7", "Sélection radio 8", "Sélection radio 9", "Sélection radio 10", "Sélection radio 11", "Sélection radio 12", "Sélection radio 13", "Sélection radio 14", "Sélection radio 15", "Sélection radio 16"}
  T4 = cluster{"START 2":dbl, "STOP 2":dbl, "CENTER 2":dbl, "SPAN 2":dbl, "CHANNEL TRACK ?":bool, "PUMP":dbl, "PROBE":dbl, "Points N° 2":i32, "SPACING 2":dbl}[]
  T5 = enum32{"No Selection", "Button 1", "Button 2", "Button 3", "Sélection radio 4", "Sélection radio 5", "Sélection radio 6", "Sélection radio 7", "Sélection radio 8", "Sélection radio 9", "Sélection radio 10", "Sélection radio 11", "Sélection radio 12", "Sélection radio 13", "Sélection radio 14", "Sélection radio 15", "Sélection radio 16"}
  T6 = cluster{"CHANNEL 1":bool, "CHANNEL 2":bool, "CHANNEL 3":bool, "CHANNEL 4":bool, "CHANNEL 5":bool, "CHANNEL 6":bool, "CHANNEL 7":bool, "CHANNEL 8":bool, "CHANNEL 9":bool, "CHANNEL 10":bool, "CHANNEL 11":bool, "CHANNEL 12":bool, "CHANNEL 13":bool, "CHANNEL 14":bool, "CHANNEL 15":bool, "CHANNEL 16":bool}
  T7 = cluster{"CHANNEL":dbl, "FREQUENCY TABLE":ext[], "MAGNITUDE TABLE":ext[], "PHASE TABLE":ext[]}
  T8 = cluster{"CHANNEL":dbl, "FREQUENCY TABLE":ext[], "MAGNITUDE TABLE":ext[], "PHASE TABLE":ext[]}[]
  T9 = cluster{"START 2":dbl, "STOP 2":dbl, "CENTER 2":dbl, "SPAN 2":dbl, "CHANNEL TRACK ?":bool, "PUMP":dbl, "PROBE":dbl, "Points N° 2":i32, "SPACING 2":dbl}
  T10 = enum16{"Freq start", "Freq stop", "Sweep size", "Decimation rate", "Freq corr", "Phase output 1", "Phase output 2", "Output level 1", "Output level 2", "GPIO", "SWEEP START"}
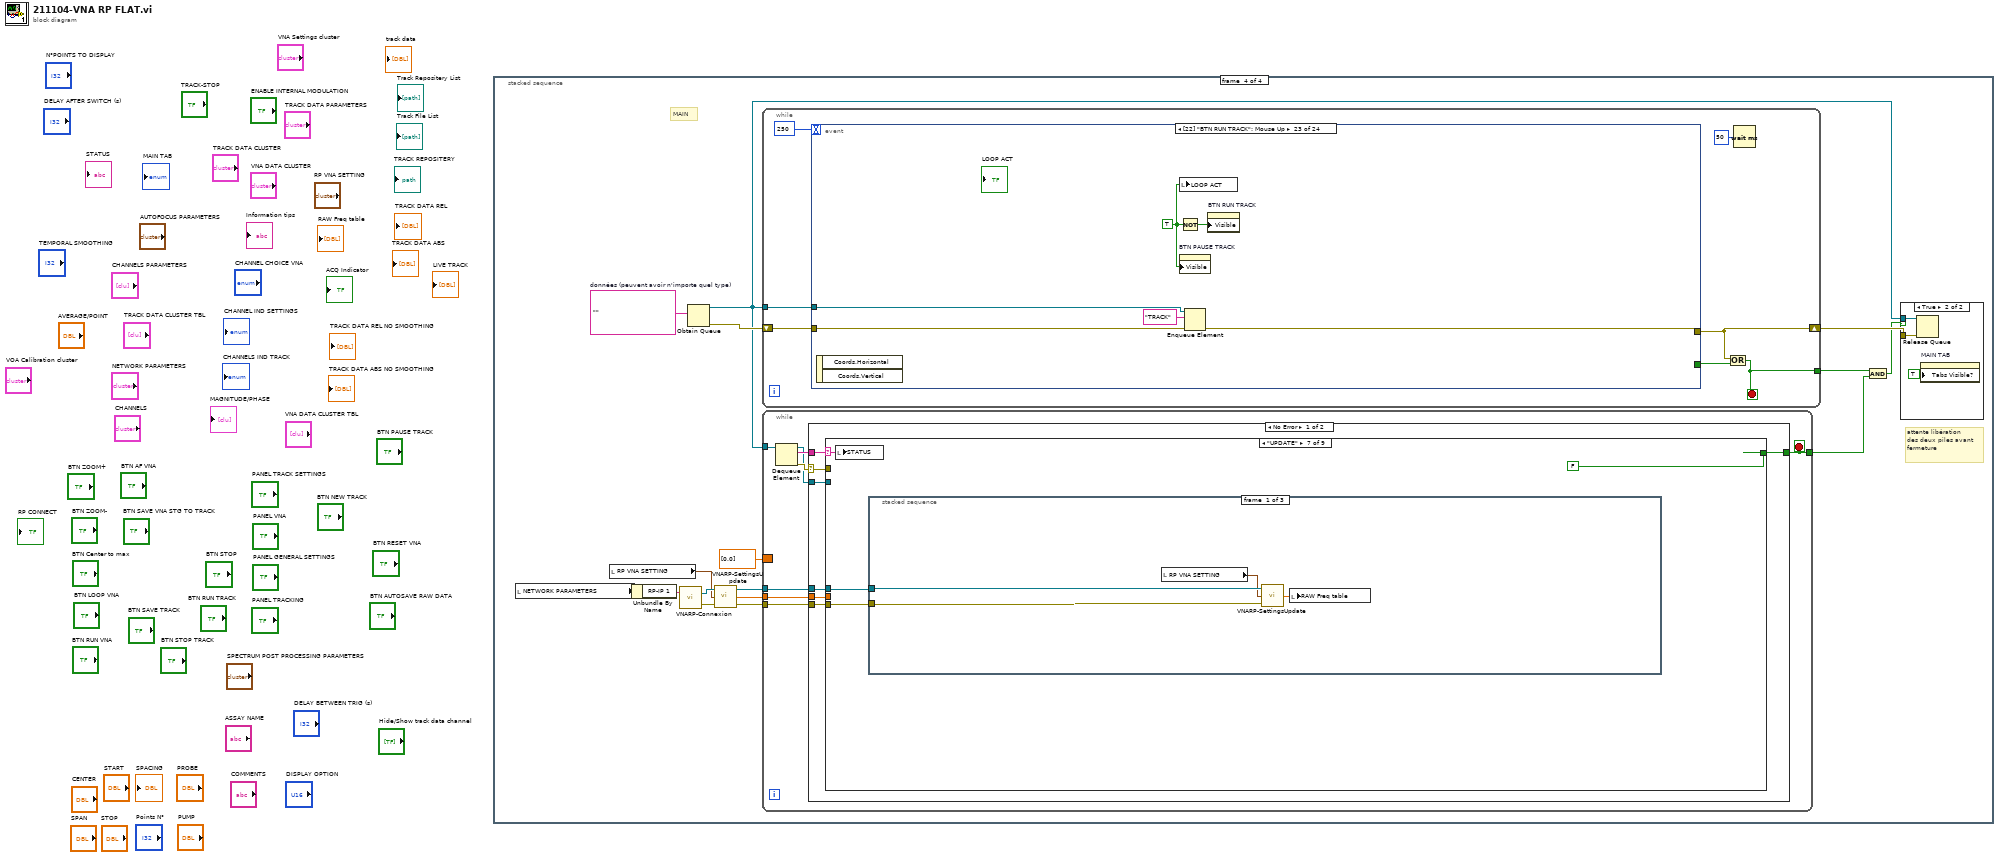
[diagram p0: block diagram]
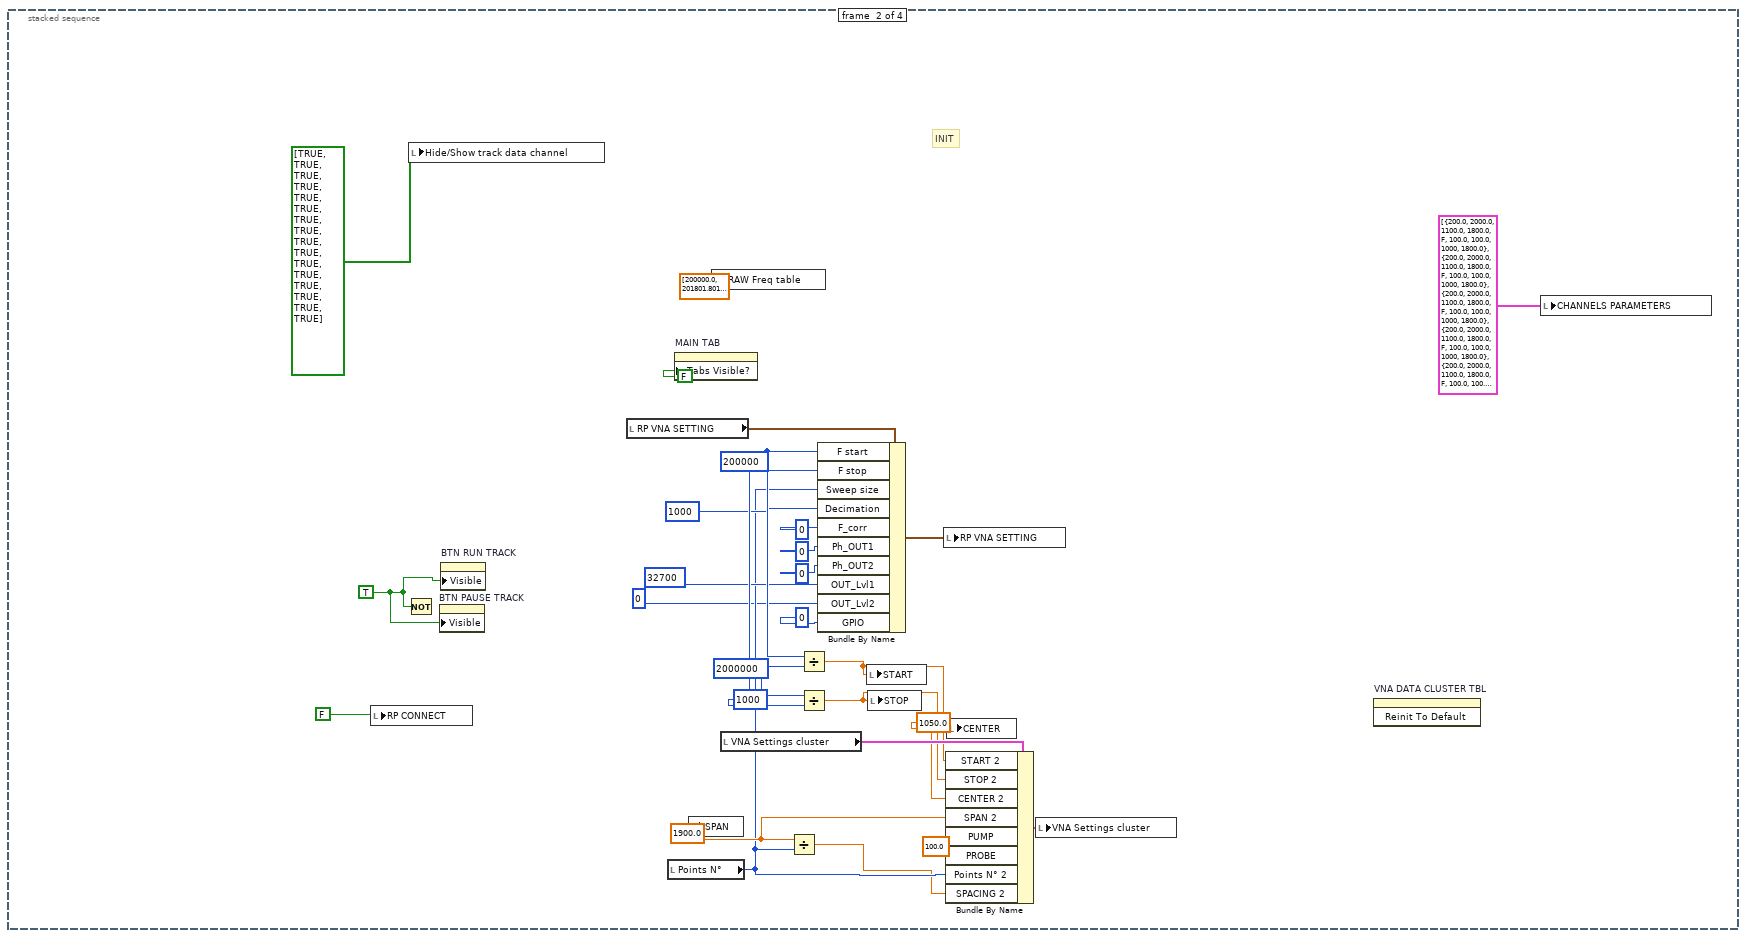
[diagram p3: hidden frame]
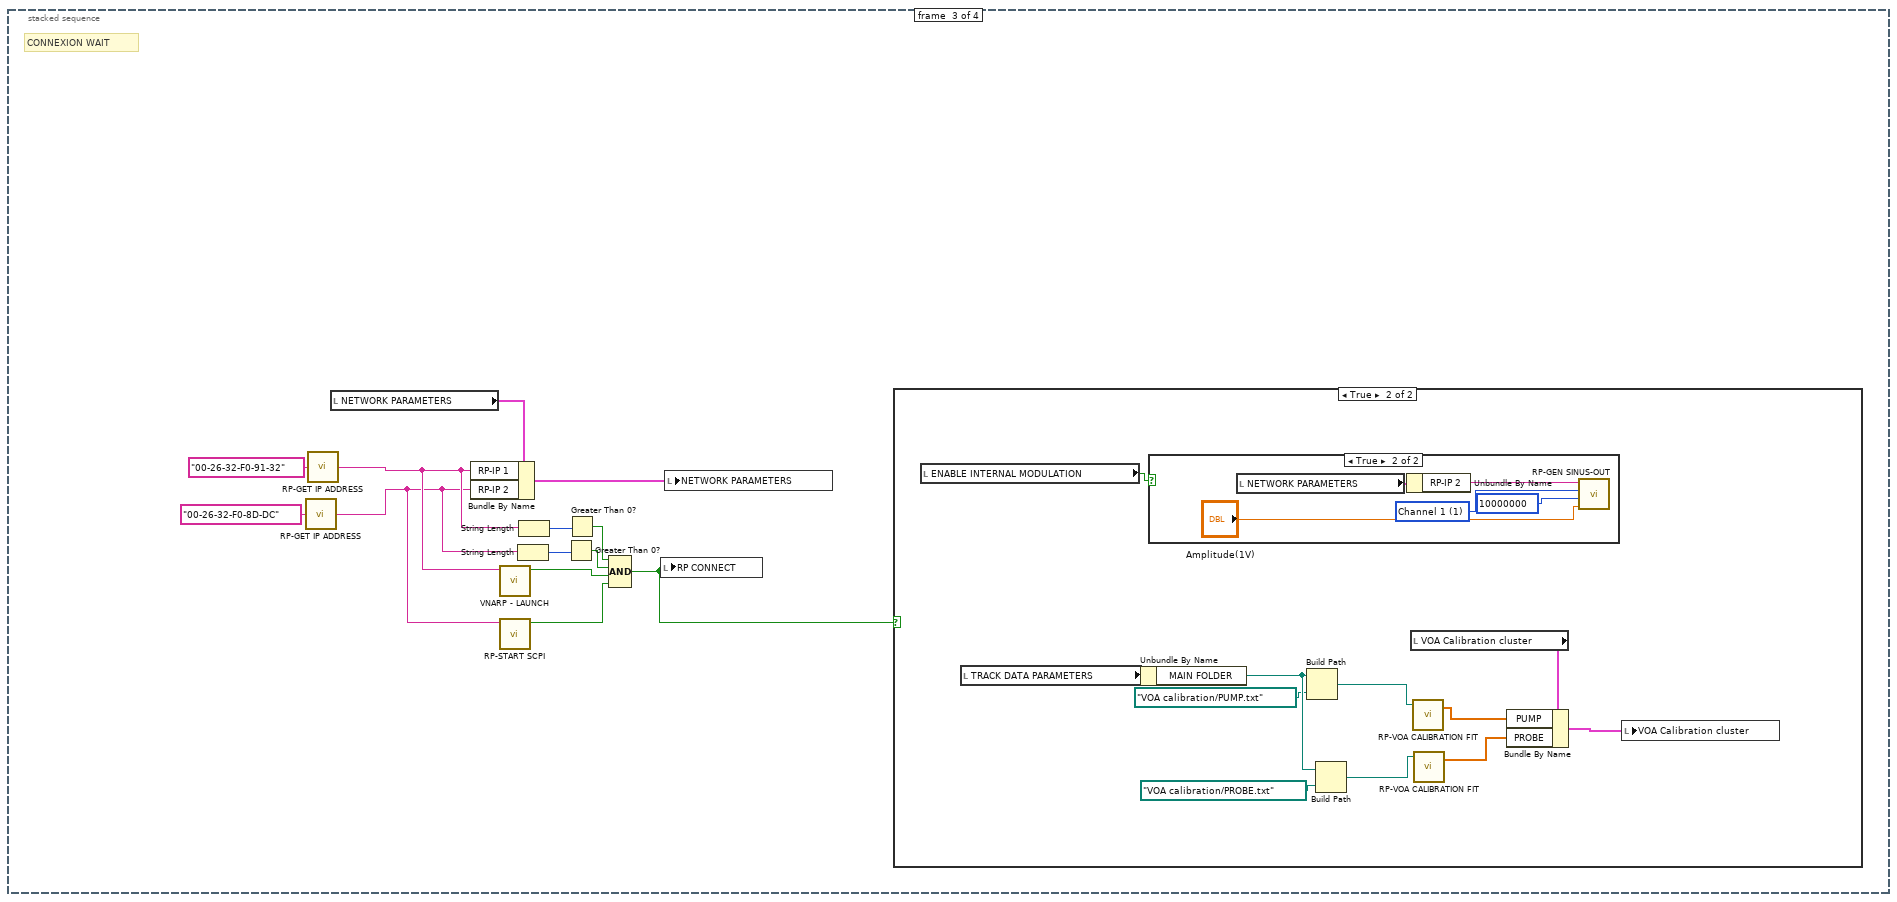
[diagram p4: hidden frame]
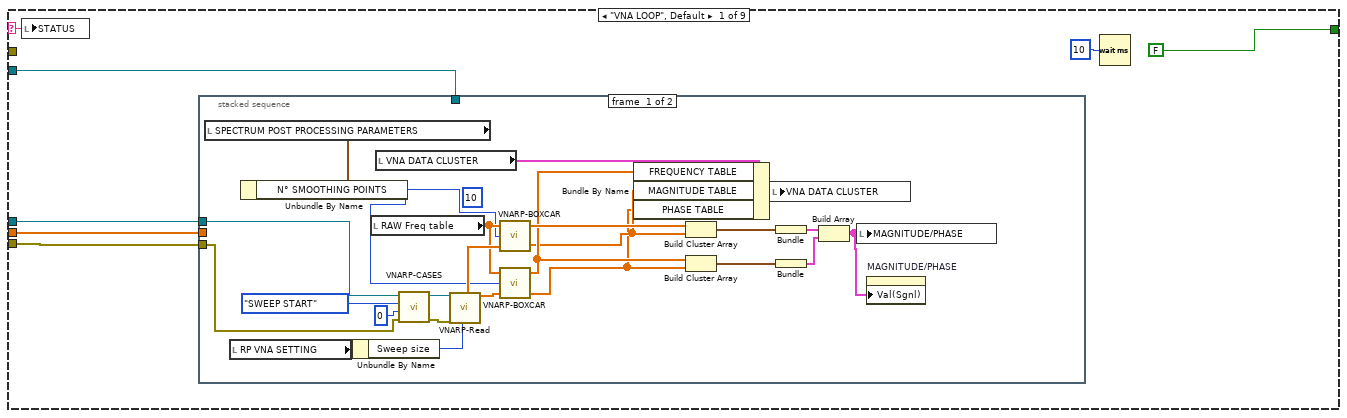
[diagram p8: hidden frame]
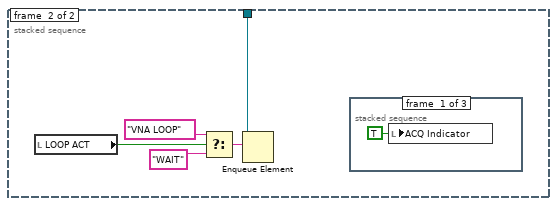
[diagram p9: hidden frame]
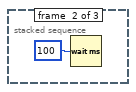
[diagram p10: hidden frame]
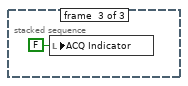
[diagram p11: hidden frame]
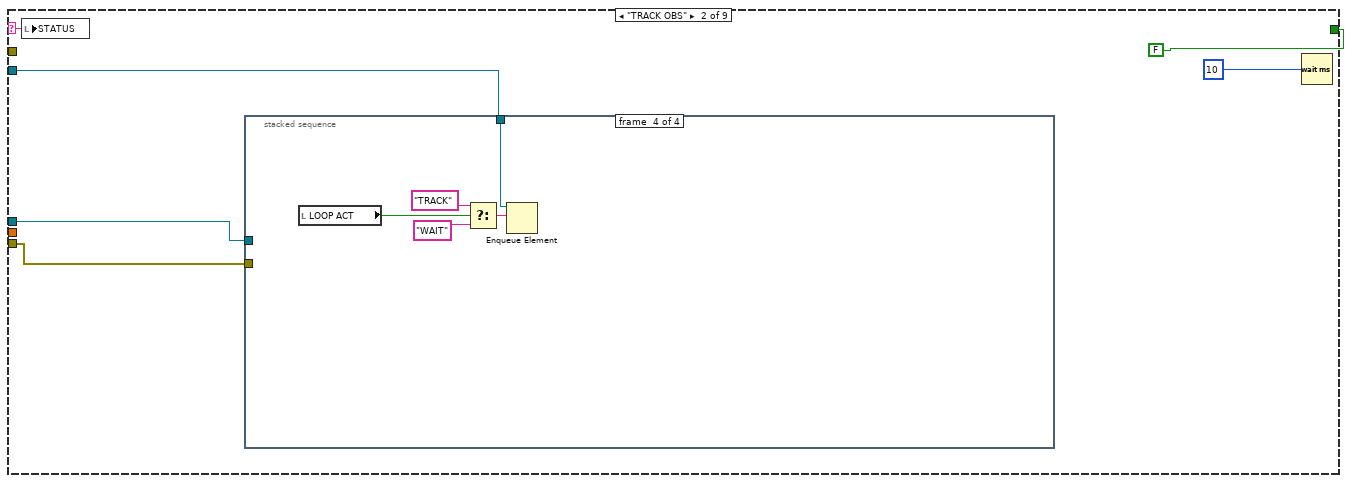
[diagram p12: hidden frame]
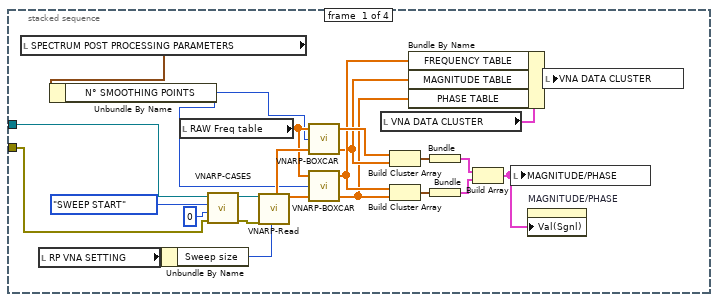
[diagram p13: hidden frame]
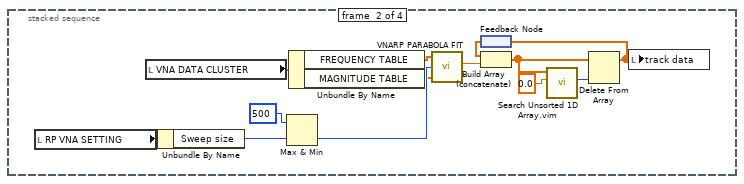
[diagram p14: hidden frame]
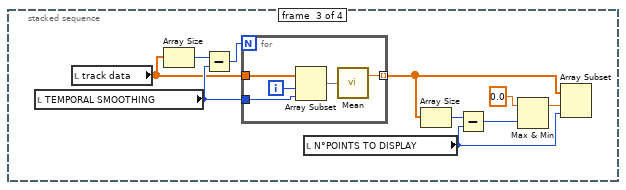
[diagram p15: hidden frame]
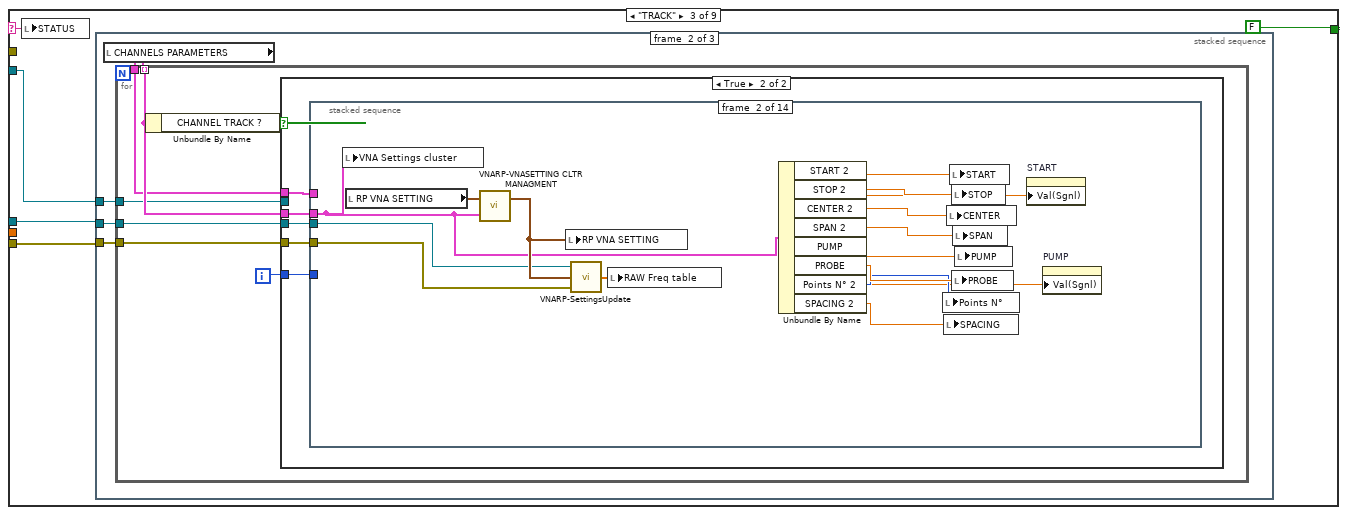
[diagram p16: hidden frame]
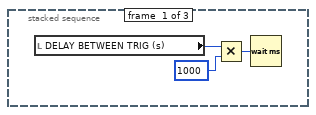
[diagram p17: hidden frame]
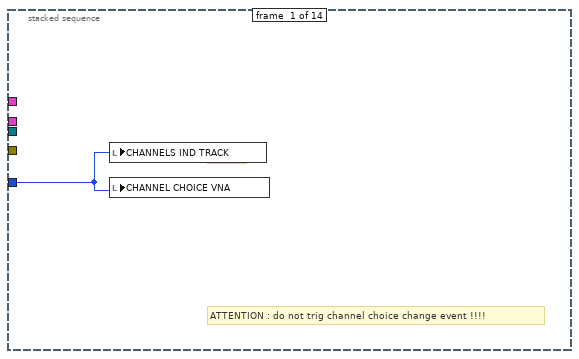
[diagram p19: hidden frame]
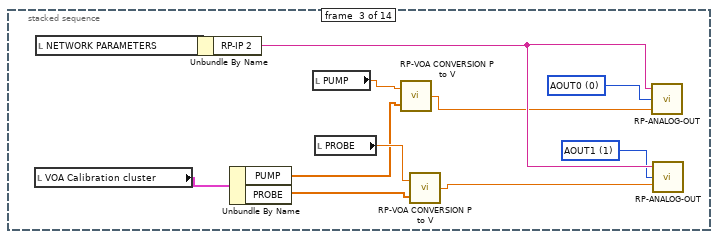
[diagram p20: hidden frame]
diagram:
  n1 = stacked-sequence {
    frame #0 {
    }
    frame #1 {
      w4 = TRUE ("x")
      w6 = 100.0 ("PUMP")
      w9 = 1900.0 ("Center")
      w10 = 1050.0 ("Center")
      w25 = u32 1000 ("Decimation")
      w23 = u32 2000000 ("Decimation")
      w24 = u32 200000 ("Decimation")
      # "INIT"
      n2 = local write "RP CONNECT"(FALSE) -> ()
      n3 = Not(x=w4) -> ()  [unwired: 1 out]
      n4 = local write "Hide/Show track data channel"(bool[] [TRUE, TRUE, TRUE, TRUE, TRUE, TRUE, TRUE, TRUE, TRUE, TRUE, TRUE, TRUE, TRUE, TRUE, TRUE, TRUE] ("Hide/Show track data channel")) -> ()
      n5 = property on="BTN PAUSE TRACK" class="Bool (strict)"("Visible"=w4) -> ()  [unwired: 2 in, 2 out]
      n6 = property on="BTN RUN TRACK" class="Bool (strict)"("Visible"=w4) -> ()  [unwired: 2 in, 2 out]
      n7 = local read "RP VNA SETTING"() -> (w27:T1)
      n8 = local read "Points N°"() -> (w8:i32)
      n9 = property on="MAIN TAB" class="TabCtl (strict)"("Tabs Visible?"=FALSE ("Onglets visibles ?")) -> ()  [unwired: 2 in, 2 out]
      n10 = local write "SPAN"(w9) -> ()
      n11 = local write "RAW Freq table"(dbl[] [200000.0, 201801.8018018018, 203603.6036036036, 205405.4054054054, 207207.20720720722, 209009.009009009, 210810.8108108108, 212612.6126126126, 214414.4144144144, 216216.2162162162, 218018.01801801802, 219819.81981981982, 221621.62162162163, 223423.42342342343, 225225.22522522524, 227027.02702702704, 228828.82882882882, 230630.63063063062, 232432.43243243243, 234234.23423423423, 236036.03603603604, 237837.83783783784, 239639.63963963964, 241441.44144144145, 243243.24324324325, 245045.04504504503, 246846.84684684683, 248648.64864864864, 250450.45045045044, 252252.25225225225, 254054.05405405405, 255855.85585585586, 257657.65765765766, 259459.45945945947, 261261.26126126124, 263063.0630630631, 264864.86486486485, 266666.6666666666, 268468.46846846846, 270270.2702702703, 272072.0720720721, 273873.87387387385, 275675.6756756757, 277477.47747747746, 279279.2792792793, 281081.08108108107, 282882.8828828829, 284684.6846846847, 286486.4864864865, 288288.2882882883, 290090.09009009006, 291891.8918918919, 293693.69369369367, 295495.4954954955, 297297.2972972973, 299099.0990990991, 300900.9009009009, 302702.7027027027, 304504.5045045045, 306306.3063063063, 308108.1081081081, 309909.90990990994, 311711.7117117117, 313513.5135135135, 315315.3153153153, 317117.1171171171, 318918.91891891893, 320720.7207207207, 322522.5225225225, 324324.3243243243, 326126.12612612615, 327927.9279279279, 329729.7297297297, 331531.53153153154, 333333.3333333333, 335135.13513513515, 336936.9369369369, 338738.7387387387, 340540.54054054053, 342342.34234234237, 344144.14414414414, 345945.9459459459, 347747.74774774775, 349549.5495495496, 351351.35135135136, 353153.15315315314, 354954.9549549549, 356756.75675675675, 358558.5585585586, 360360.36036036036, 362162.16216216213, 363963.96396396396, 365765.7657657658, 367567.5675675676, 369369.36936936935, 371171.1711711711, 372972.97297297296, 374774.7747747748, 376576.57657657657, 378378.37837837834, 380180.1801801802, 381981.981981982, 383783.7837837838, 385585.58558558556, 387387.38738738734, 389189.1891891892, 390990.990990991, 392792.7927927928, 394594.59459459456, 396396.3963963964, 398198.1981981982, 400000.0, 401801.8018018018, 403603.6036036036, 405405.4054054054, 407207.2072072072, 409009.009009009, 410810.81081081077, 412612.6126126126, 414414.41441441444, 416216.2162162162, 418018.018018018, 419819.8198198198, 421621.62162162166, 423423.42342342343, 425225.2252252252, 427027.027027027, 428828.8288288288, 430630.63063063065, 432432.4324324324, 434234.2342342342, 436036.03603603604, 437837.83783783787, 439639.63963963964, 441441.4414414414, 443243.2432432432, 445045.04504504503, 446846.84684684686, 448648.64864864864, 450450.4504504504, 452252.25225225225, 454054.0540540541, 455855.85585585586, 457657.65765765763, 459459.4594594594, 461261.26126126124, 463063.0630630631, 464864.86486486485, 466666.6666666666, 468468.46846846846, 470270.27027027024, 472072.0720720721, 473873.87387387385, 475675.6756756757, 477477.47747747746, 479279.2792792793, 481081.08108108107, 482882.8828828829, 484684.6846846847, 486486.48648648645, 488288.2882882883, 490090.09009009006, 491891.8918918919, 493693.69369369367, 495495.4954954955, 497297.2972972973, 499099.0990990991, 500900.9009009009, 502702.70270270266, 504504.5045045045, 506306.3063063063, 508108.1081081081, 509909.9099099099, 511711.7117117117, 513513.5135135135, 515315.3153153153, 517117.1171171171, 518918.91891891893, 520720.7207207207, 522522.5225225225, 524324.3243243243, 526126.1261261262, 527927.9279279279, 529729.7297297297, 531531.5315315316, 533333.3333333333, 535135.1351351351, 536936.9369369369, 538738.7387387387, 540540.5405405406, 542342.3423423423, 544144.1441441441, 545945.9459459459, 547747.7477477477, 549549.5495495496, 551351.3513513514, 553153.1531531531, 554954.9549549549, 556756.7567567567, 558558.5585585586, 560360.3603603604, 562162.1621621621, 563963.963963964, 565765.7657657657, 567567.5675675676, 569369.3693693693, 571171.1711711711, 572972.972972973, 574774.7747747747, 576576.5765765766, 578378.3783783783, 580180.1801801801, 581981.981981982, 583783.7837837838, 585585.5855855856, 587387.3873873875, 589189.1891891891, 590990.990990991, 592792.7927927928, 594594.5945945946, 596396.3963963964, 598198.1981981981, 600000.0, 601801.8018018018, 603603.6036036036, 605405.4054054054, 607207.2072072072, 609009.009009009, 610810.8108108108, 612612.6126126125, 614414.4144144144, 616216.2162162162, 618018.018018018, 619819.8198198199, 621621.6216216215, 623423.4234234234, 625225.2252252252, 627027.027027027, 628828.8288288289, 630630.6306306305, 632432.4324324324, 634234.2342342342, 636036.036036036, 637837.8378378379, 639639.6396396396, 641441.4414414414, 643243.2432432433, 645045.045045045, 646846.8468468469, 648648.6486486486, 650450.4504504504, 652252.2522522523, 654054.054054054, 655855.8558558559, 657657.6576576576, 659459.4594594594, 661261.2612612613, 663063.063063063, 664864.8648648649, 666666.6666666666, 668468.4684684684, 670270.2702702703, 672072.0720720721, 673873.8738738738, 675675.6756756757, 677477.4774774774, 679279.2792792793, 681081.0810810811, 682882.8828828828, 684684.6846846847, 686486.4864864864, 688288.2882882883, 690090.0900900901, 691891.8918918918, 693693.6936936937, 695495.4954954955, 697297.2972972973, 699099.099099099, 700900.9009009008, 702702.7027027027, 704504.5045045045, 706306.3063063063, 708108.1081081082, 709909.9099099098, 711711.7117117117, 713513.5135135135, 715315.3153153153, 717117.1171171172, 718918.9189189188, 720720.7207207207, 722522.5225225225, 724324.3243243243, 726126.1261261262, 727927.9279279279, 729729.7297297297, 731531.5315315315, 733333.3333333333, 735135.1351351351, 736936.9369369369, 738738.7387387387, 740540.5405405405, 742342.3423423424, 744144.1441441441, 745945.9459459459, 747747.7477477477, 749549.5495495496, 751351.3513513514, 753153.1531531531, 754954.9549549549, 756756.7567567567, 758558.5585585586, 760360.3603603604, 762162.1621621621, 763963.9639639639, 765765.7657657658, 767567.5675675676, 769369.3693693693, 771171.1711711711, 772972.9729729729, 774774.7747747748, 776576.5765765766, 778378.3783783783, 780180.1801801801, 781981.981981982, 783783.7837837838, 785585.5855855856, 787387.3873873873, 789189.1891891891, 790990.990990991, 792792.7927927928, 794594.5945945946, 796396.3963963963, 798198.1981981982, 800000.0, 801801.8018018018, 803603.6036036036, 805405.4054054053, 807207.2072072072, 809009.009009009, 810810.8108108108, 812612.6126126125, 814414.4144144144, 816216.2162162162, 818018.018018018, 819819.8198198198, 821621.6216216215, 823423.4234234234, 825225.2252252252, 827027.027027027, 828828.8288288288, 830630.6306306307, 832432.4324324324, 834234.2342342342, 836036.036036036, 837837.8378378379, 839639.6396396396, 841441.4414414414, 843243.2432432432, 845045.045045045, 846846.8468468469, 848648.6486486486, 850450.4504504504, 852252.2522522522, 854054.0540540541, 855855.8558558559, 857657.6576576576, 859459.4594594594, 861261.2612612612, 863063.0630630631, 864864.8648648649, 866666.6666666666, 868468.4684684684, 870270.2702702703, 872072.0720720721, 873873.8738738738, 875675.6756756756, 877477.4774774774, 879279.2792792793, 881081.0810810811, 882882.8828828828, 884684.6846846846, 886486.4864864865, 888288.2882882883, 890090.0900900901, 891891.8918918918, 893693.6936936936, 895495.4954954955, 897297.2972972973, 899099.099099099, 900900.9009009008, 902702.7027027027, 904504.5045045045, 906306.3063063063, 908108.108108108, 909909.9099099098, 911711.7117117117, 913513.5135135135, 915315.3153153153, 917117.117117117, 918918.9189189189, 920720.7207207207, 922522.5225225225, 924324.3243243243, 926126.1261261262, 927927.9279279279, 929729.7297297297, 931531.5315315315, 933333.3333333333, 935135.1351351351, 936936.9369369369, 938738.7387387387, 940540.5405405405, 942342.3423423424, 944144.1441441441, 945945.9459459459, 947747.7477477477, 949549.5495495495, 951351.3513513514, 953153.1531531531, 954954.9549549549, 956756.7567567567, 958558.5585585586, 960360.3603603604, 962162.1621621621, 963963.9639639639, 965765.7657657657, 967567.5675675676, 969369.3693693693, 971171.1711711711, 972972.9729729729, 974774.7747747748, 976576.5765765766, 978378.3783783783, 980180.1801801801, 981981.9819819819, 983783.7837837838, 985585.5855855856, 987387.3873873873, 989189.1891891891, 990990.990990991, 992792.7927927928, 994594.5945945946, 996396.3963963963, 998198.1981981982, 1000000.0, 1001801.8018018018, 1003603.6036036036, 1005405.4054054053, 1007207.2072072072, 1009009.009009009, 1010810.8108108108, 1012612.6126126125, 1014414.4144144144, 1016216.2162162162, 1018018.018018018, 1019819.8198198198, 1021621.6216216215, 1023423.4234234234, 1025225.2252252252, 1027027.027027027, 1028828.8288288288, 1030630.6306306307, 1032432.4324324324, 1034234.2342342342, 1036036.036036036, 1037837.8378378378, 1039639.6396396396, 1041441.4414414414, 1043243.2432432432, 1045045.045045045, 1046846.8468468469, 1048648.6486486485, 1050450.4504504504, 1052252.2522522523, 1054054.054054054, 1055855.8558558559, 1057657.6576576577, 1059459.4594594594, 1061261.261261261, 1063063.0630630632, 1064864.8648648649, 1066666.6666666665, 1068468.4684684684, 1070270.2702702703, 1072072.072072072, 1073873.8738738738, 1075675.6756756757, 1077477.4774774774, 1079279.2792792793, 1081081.0810810812, 1082882.8828828828, 1084684.6846846845, 1086486.4864864866, 1088288.2882882883, 1090090.09009009, 1091891.8918918918, 1093693.6936936937, 1095495.4954954954, 1097297.2972972973, 1099099.0990990992, 1100900.9009009008, 1102702.7027027027, 1104504.5045045046, 1106306.3063063063, 1108108.108108108, 1109909.9099099098, 1111711.7117117117, 1113513.5135135134, 1115315.3153153153, 1117117.1171171172, 1118918.9189189188, 1120720.7207207207, 1122522.5225225226, 1124324.3243243243, 1126126.126126126, 1127927.927927928, 1129729.7297297297, 1131531.5315315314, 1133333.3333333333, 1135135.1351351351, 1136936.9369369368, 1138738.7387387387, 1140540.5405405406, 1142342.3423423423, 1144144.1441441441, 1145945.945945946, 1147747.7477477477, 1149549.5495495494, 1151351.3513513515, 1153153.1531531531, 1154954.9549549548, 1156756.7567567567, 1158558.5585585586, 1160360.3603603602, 1162162.1621621621, 1163963.963963964, 1165765.7657657657, 1167567.5675675676, 1169369.3693693695, 1171171.1711711711, 1172972.9729729728, 1174774.774774775, 1176576.5765765766, 1178378.3783783782, 1180180.1801801801, 1181981.981981982, 1183783.7837837837, 1185585.5855855856, 1187387.3873873875, 1189189.189189189, 1190990.990990991, 1192792.792792793, 1194594.5945945946, 1196396.3963963962, 1198198.198198198, 1200000.0, 1201801.8018018017, 1203603.6036036036, 1205405.4054054054, 1207207.207207207, 1209009.009009009, 1210810.810810811, 1212612.6126126125, 1214414.4144144142, 1216216.2162162163, 1218018.018018018, 1219819.8198198196, 1221621.6216216215, 1223423.4234234234, 1225225.225225225, 1227027.027027027, 1228828.8288288289, 1230630.6306306305, 1232432.4324324324, 1234234.2342342343, 1236036.036036036, 1237837.8378378376, 1239639.6396396398, 1241441.4414414414, 1243243.243243243, 1245045.045045045, 1246846.8468468469, 1248648.6486486485, 1250450.4504504504, 1252252.2522522523, 1254054.054054054, 1255855.8558558559, 1257657.6576576575, 1259459.4594594594, 1261261.2612612613, 1263063.063063063, 1264864.8648648649, 1266666.6666666665, 1268468.4684684684, 1270270.2702702703, 1272072.072072072, 1273873.8738738738, 1275675.6756756757, 1277477.4774774774, 1279279.2792792793, 1281081.081081081, 1282882.8828828828, 1284684.6846846847, 1286486.4864864864, 1288288.2882882883, 1290090.09009009, 1291891.8918918918, 1293693.6936936937, 1295495.4954954954, 1297297.2972972973, 1299099.0990990992, 1300900.9009009008, 1302702.7027027027, 1304504.5045045044, 1306306.3063063063, 1308108.1081081082, 1309909.9099099098, 1311711.7117117117, 1313513.5135135134, 1315315.3153153153, 1317117.1171171172, 1318918.9189189188, 1320720.7207207207, 1322522.5225225224, 1324324.3243243243, 1326126.1261261262, 1327927.9279279278, 1329729.7297297297, 1331531.5315315316, 1333333.3333333333, 1335135.1351351351, 1336936.9369369368, 1338738.7387387387, 1340540.5405405406, 1342342.3423423423, 1344144.1441441441, 1345945.9459459458, 1347747.7477477477, 1349549.5495495496, 1351351.3513513512, 1353153.1531531531, 1354954.9549549548, 1356756.7567567567, 1358558.5585585586, 1360360.3603603602, 1362162.1621621621, 1363963.963963964, 1365765.7657657657, 1367567.5675675676, 1369369.3693693692, 1371171.1711711711, 1372972.972972973, 1374774.7747747747, 1376576.5765765766, 1378378.3783783782, 1380180.1801801801, 1381981.981981982, 1383783.7837837837, 1385585.5855855856, 1387387.3873873875, 1389189.189189189, 1390990.990990991, 1392792.7927927927, 1394594.5945945946, 1396396.3963963964, 1398198.198198198, 1400000.0, 1401801.8018018017, 1403603.6036036036, 1405405.4054054054, 1407207.207207207, 1409009.009009009, 1410810.8108108107, 1412612.6126126125, 1414414.4144144144, 1416216.216216216, 1418018.018018018, 1419819.8198198199, 1421621.6216216215, 1423423.4234234234, 1425225.225225225, 1427027.027027027, 1428828.8288288289, 1430630.6306306305, 1432432.4324324324, 1434234.234234234, 1436036.036036036, 1437837.8378378379, 1439639.6396396395, 1441441.4414414414, 1443243.243243243, 1445045.045045045, 1446846.8468468469, 1448648.6486486485, 1450450.4504504504, 1452252.2522522523, 1454054.054054054, 1455855.8558558559, 1457657.6576576575, 1459459.4594594594, 1461261.2612612613, 1463063.063063063, 1464864.8648648649, 1466666.6666666665, 1468468.4684684684, 1470270.2702702703, 1472072.072072072, 1473873.8738738738, 1475675.6756756757, 1477477.4774774774, 1479279.2792792793, 1481081.081081081, 1482882.8828828828, 1484684.6846846847, 1486486.4864864864, 1488288.2882882883, 1490090.09009009, 1491891.8918918918, 1493693.6936936937, 1495495.4954954954, 1497297.2972972973, 1499099.099099099, 1500900.9009009008, 1502702.7027027027, 1504504.5045045044, 1506306.3063063063, 1508108.1081081082, 1509909.9099099098, 1511711.7117117117, 1513513.5135135134, 1515315.3153153153, 1517117.1171171172, 1518918.9189189188, 1520720.7207207207, 1522522.5225225224, 1524324.3243243243, 1526126.1261261262, 1527927.9279279278, 1529729.7297297297, 1531531.5315315314, 1533333.3333333333, 1535135.1351351351, 1536936.9369369368, 1538738.7387387387, 1540540.5405405406, 1542342.3423423423, 1544144.1441441441, 1545945.9459459458, 1547747.7477477477, 1549549.5495495496, 1551351.3513513512, 1553153.1531531531, 1554954.9549549548, 1556756.7567567567, 1558558.5585585586, 1560360.3603603602, 1562162.1621621621, 1563963.963963964, 1565765.7657657657, 1567567.5675675676, 1569369.3693693692, 1571171.1711711711, 1572972.972972973, 1574774.7747747747, 1576576.5765765766, 1578378.3783783782, 1580180.1801801801, 1581981.981981982, 1583783.7837837837, 1585585.5855855856, 1587387.3873873872, 1589189.189189189, 1590990.990990991, 1592792.7927927927, 1594594.5945945946, 1596396.3963963964, 1598198.198198198, 1600000.0, 1601801.8018018017, 1603603.6036036036, 1605405.4054054054, 1607207.207207207, 1609009.009009009, 1610810.8108108107, 1612612.6126126125, 1614414.4144144144, 1616216.216216216, 1618018.018018018, 1619819.8198198196, 1621621.6216216215, 1623423.4234234234, 1625225.225225225, 1627027.027027027, 1628828.8288288289, 1630630.6306306305, 1632432.4324324324, 1634234.234234234, 1636036.036036036, 1637837.8378378379, 1639639.6396396395, 1641441.4414414414, 1643243.243243243, 1645045.045045045, 1646846.8468468469, 1648648.6486486485, 1650450.4504504504, 1652252.2522522523, 1654054.054054054, 1655855.8558558559, 1657657.6576576575, 1659459.4594594594, 1661261.2612612613, 1663063.063063063, 1664864.8648648649, 1666666.6666666665, 1668468.4684684684, 1670270.2702702703, 1672072.072072072, 1673873.8738738738, 1675675.6756756755, 1677477.4774774774, 1679279.2792792793, 1681081.081081081, 1682882.8828828828, 1684684.6846846847, 1686486.4864864864, 1688288.2882882883, 1690090.09009009, 1691891.8918918918, 1693693.6936936937, 1695495.4954954954, 1697297.2972972973, 1699099.099099099, 1700900.9009009008, 1702702.7027027027, 1704504.5045045044, 1706306.3063063063, 1708108.108108108, 1709909.9099099098, 1711711.7117117117, 1713513.5135135134, 1715315.3153153153, 1717117.1171171172, 1718918.9189189188, 1720720.7207207207, 1722522.5225225224, 1724324.3243243243, 1726126.1261261262, 1727927.9279279278, 1729729.7297297297, 1731531.5315315314, 1733333.3333333333, 1735135.1351351351, 1736936.9369369368, 1738738.7387387387, 1740540.5405405406, 1742342.3423423423, 1744144.1441441441, 1745945.9459459458, 1747747.7477477477, 1749549.5495495496, 1751351.3513513512, 1753153.1531531531, 1754954.9549549548, 1756756.7567567567, 1758558.5585585586, 1760360.3603603602, 1762162.1621621621, 1763963.9639639638, 1765765.7657657657, 1767567.5675675676, 1769369.3693693692, 1771171.1711711711, 1772972.972972973, 1774774.7747747747, 1776576.5765765766, 1778378.3783783782, 1780180.1801801801, 1781981.981981982, 1783783.7837837837, 1785585.5855855856, 1787387.3873873872, 1789189.189189189, 1790990.990990991, 1792792.7927927927, 1794594.5945945946, 1796396.3963963964, 1798198.198198198, 1800000.0, 1801801.8018018017, 1803603.6036036036, 1805405.4054054054, 1807207.207207207, 1809009.009009009, 1810810.8108108107, 1812612.6126126125, 1814414.4144144144, 1816216.216216216, 1818018.018018018, 1819819.8198198196, 1821621.6216216215, 1823423.4234234234, 1825225.225225225, 1827027.027027027, 1828828.8288288289, 1830630.6306306305, 1832432.4324324324, 1834234.234234234, 1836036.036036036, 1837837.8378378379, 1839639.6396396395, 1841441.4414414414, 1843243.243243243, 1845045.045045045, 1846846.8468468469, 1848648.6486486485, 1850450.4504504504, 1852252.252252252, 1854054.054054054, 1855855.8558558559, 1857657.6576576575, 1859459.4594594594, 1861261.2612612613, 1863063.063063063, 1864864.8648648649, 1866666.6666666665, 1868468.4684684684, 1870270.2702702703, 1872072.072072072, 1873873.8738738738, 1875675.6756756755, 1877477.4774774774, 1879279.2792792793, 1881081.081081081, 1882882.8828828828, 1884684.6846846847, 1886486.4864864864, 1888288.2882882883, 1890090.09009009, 1891891.8918918918, 1893693.6936936937, 1895495.4954954954, 1897297.2972972973, 1899099.099099099, 1900900.9009009008, 1902702.7027027027, 1904504.5045045044, 1906306.3063063063, 1908108.108108108, 1909909.9099099098, 1911711.7117117117, 1913513.5135135134, 1915315.3153153153, 1917117.1171171172, 1918918.9189189188, 1920720.7207207207, 1922522.5225225224, 1924324.3243243243, 1926126.1261261262, 1927927.9279279278, 1929729.7297297297, 1931531.5315315314, 1933333.3333333333, 1935135.1351351351, 1936936.9369369368, 1938738.7387387387, 1940540.5405405404, 1942342.3423423423, 1944144.1441441441, 1945945.9459459458, 1947747.7477477477, 1949549.5495495496, 1951351.3513513512, 1953153.1531531531, 1954954.9549549548, 1956756.7567567567, 1958558.5585585586, 1960360.3603603602, 1962162.1621621621, 1963963.9639639638, 1965765.7657657657, 1967567.5675675676, 1969369.3693693692, 1971171.1711711711, 1972972.972972973, 1974774.7747747747, 1976576.5765765766, 1978378.3783783782, 1980180.1801801801, 1981981.981981982, 1983783.7837837837, 1985585.5855855856, 1987387.3873873872, 1989189.189189189, 1990990.990990991, 1992792.7927927927, 1994594.5945945946, 1996396.3963963962, 1998198.198198198, 2000000.0] ("RAW Freq table")) -> ()
      n12 = local read "VNA Settings cluster"() -> (w14:T9)
      n13 = Divide(x=w9, y=w8) -> (x/y=w7:dbl)
      n14 = Divide(x=w24, y=w25) -> (x/y=w11:dbl)
      n15 = Divide(x=w23, y=w25) -> (x/y=w12:dbl)
      n16 = Bundle By Name(cluster=w27, "F start"=w24, "F stop"=w23, "Sweep size"=w8, "Decimation"=u32 1000, "F_corr"=u32 0, "Ph_OUT1"=u32 0, "Ph_OUT2"=u32 0 ("F_corr"), "OUT_Lvl1"=u32 32700 ("F_corr"), "OUT_Lvl2"=u32 0 ("F_corr"), "GPIO"=u32 0 ("F_corr")) -> (w26:T1)
      n17 = local write "START"(w11) -> ()
      n18 = local write "STOP"(w12) -> ()
      n19 = local write "RP VNA SETTING"(w26) -> ()
      n20 = Bundle By Name(cluster=w14, "START 2"=w11, "STOP 2"=w12, "CENTER 2"=w10, "SPAN 2"=w9, "PUMP"=w6, "PROBE"=w6, "Points N° 2"=w8, "SPACING 2"=w7) -> (w13:T9)
      n21 = local write "CENTER"(w10) -> ()
      n22 = local write "VNA Settings cluster"(w13) -> ()
      n23 = invoke on="VNA DATA CLUSTER TBL" class="Arr (strict)" method="Reinit To Default"() -> ()  [unwired: 3 in, 3 out]
      n24 = local write "CHANNELS PARAMETERS"(T4 [{"START 2"=200.0, "STOP 2"=2000.0, "CENTER 2"=1100.0, "SPAN 2"=1800.0, "CHANNEL TRACK ?"=FALSE, "PUMP"=100.0, "PROBE"=100.0, "Points N° 2"=1000, "SPACING 2"=1800.0}, {"START 2"=200.0, "STOP 2"=2000.0, "CENTER 2"=1100.0, "SPAN 2"=1800.0, "CHANNEL TRACK ?"=FALSE, "PUMP"=100.0, "PROBE"=100.0, "Points N° 2"=1000, "SPACING 2"=1800.0}, {"START 2"=200.0, "STOP 2"=2000.0, "CENTER 2"=1100.0, "SPAN 2"=1800.0, "CHANNEL TRACK ?"=FALSE, "PUMP"=100.0, "PROBE"=100.0, "Points N° 2"=1000, "SPACING 2"=1800.0}, {"START 2"=200.0, "STOP 2"=2000.0, "CENTER 2"=1100.0, "SPAN 2"=1800.0, "CHANNEL TRACK ?"=FALSE, "PUMP"=100.0, "PROBE"=100.0, "Points N° 2"=1000, "SPACING 2"=1800.0}, {"START 2"=200.0, "STOP 2"=2000.0, "CENTER 2"=1100.0, "SPAN 2"=1800.0, "CHANNEL TRACK ?"=FALSE, "PUMP"=100.0, "PROBE"=100.0, "Points N° 2"=1000, "SPACING 2"=1800.0}, {"START 2"=200.0, "STOP 2"=2000.0, "CENTER 2"=1100.0, "SPAN 2"=1800.0, "CHANNEL TRACK ?"=FALSE, "PUMP"=100.0, "PROBE"=100.0, "Points N° 2"=1000, "SPACING 2"=1800.0}, {"START 2"=200.0, "STOP 2"=2000.0, "CENTER 2"=1100.0, "SPAN 2"=1800.0, "CHANNEL TRACK ?"=FALSE, "PUMP"=100.0, "PROBE"=100.0, "Points N° 2"=1000, "SPACING 2"=1800.0}, {"START 2"=200.0, "STOP 2"=2000.0, "CENTER 2"=1100.0, "SPAN 2"=1800.0, "CHANNEL TRACK ?"=FALSE, "PUMP"=100.0, "PROBE"=100.0, "Points N° 2"=1000, "SPACING 2"=1800.0}, {"START 2"=200.0, "STOP 2"=2000.0, "CENTER 2"=1100.0, "SPAN 2"=1800.0, "CHANNEL TRACK ?"=FALSE, "PUMP"=100.0, "PROBE"=100.0, "Points N° 2"=1000, "SPACING 2"=1800.0}, {"START 2"=200.0, "STOP 2"=2000.0, "CENTER 2"=1100.0, "SPAN 2"=1800.0, "CHANNEL TRACK ?"=FALSE, "PUMP"=100.0, "PROBE"=100.0, "Points N° 2"=1000, "SPACING 2"=1800.0}, {"START 2"=200.0, "STOP 2"=2000.0, "CENTER 2"=1100.0, "SPAN 2"=1800.0, "CHANNEL TRACK ?"=FALSE, "PUMP"=100.0, "PROBE"=100.0, "Points N° 2"=1000, "SPACING 2"=1800.0}, {"START 2"=200.0, "STOP 2"=2000.0, "CENTER 2"=1100.0, "SPAN 2"=1800.0, "CHANNEL TRACK ?"=FALSE, "PUMP"=100.0, "PROBE"=100.0, "Points N° 2"=1000, "SPACING 2"=1800.0}, {"START 2"=200.0, "STOP 2"=2000.0, "CENTER 2"=1100.0, "SPAN 2"=1800.0, "CHANNEL TRACK ?"=FALSE, "PUMP"=100.0, "PROBE"=100.0, "Points N° 2"=1000, "SPACING 2"=1800.0}, {"START 2"=200.0, "STOP 2"=2000.0, "CENTER 2"=1100.0, "SPAN 2"=1800.0, "CHANNEL TRACK ?"=FALSE, "PUMP"=100.0, "PROBE"=100.0, "Points N° 2"=1000, "SPACING 2"=1800.0}, {"START 2"=200.0, "STOP 2"=2000.0, "CENTER 2"=1100.0, "SPAN 2"=1800.0, "CHANNEL TRACK ?"=FALSE, "PUMP"=100.0, "PROBE"=100.0, "Points N° 2"=1000, "SPACING 2"=1800.0}, {"START 2"=200.0, "STOP 2"=2000.0, "CENTER 2"=1100.0, "SPAN 2"=1800.0, "CHANNEL TRACK ?"=FALSE, "PUMP"=100.0, "PROBE"=100.0, "Points N° 2"=1000, "SPACING 2"=1800.0}] ("CHANNELS PARAMETERS")) -> ()
    }
    frame #2 {
      # "CONNEXION WAIT"
      n25 = call "RP-GET IP ADDRESS.vi"("MAC address"="00-26-32-F0-8D-DC") -> ("IP address"=w29:string)
      n26 = call "RP-GET IP ADDRESS.vi"("MAC address"="00-26-32-F0-91-32") -> ("IP address"=w35:string)
      n27 = local read "NETWORK PARAMETERS"() -> (w40:cluster{"RP-IP 1":string, "RP-IP 2":string})
      n28 = Bundle By Name(cluster=w40, "RP-IP 1"=w35, "RP-IP 2"=w29) -> (w39:cluster{"RP-IP 1":string, "RP-IP 2":string})
      n29 = call "VNARP - LAUNCH.vi"("RP IP"=w35) -> ("VNA launched ?"=w36:bool)  [unwired: 10 in]
      n30 = call "RP-START SCPI.vi"("RP IP"=w29) -> ("SCPI launched ?"=w28:bool)  [unwired: 10 in]
      n31 = String Length(string=w29) -> (length=w38:i32)
      n32 = String Length(string=w35) -> (length=w37:i32)
      n33 = Greater Than 0?(x=w38) -> (x > 0?=w33:bool)
      n34 = Greater Than 0?(x=w37) -> (x > 0?=w34:bool)
      n35 = Compound Arithmetic op=AND(w34, w33, w36, w28) -> (w30:bool)
      n36 = local write "RP CONNECT"(w30) -> ()
      n37 = local write "NETWORK PARAMETERS"(w39) -> ()
      n38 = case shown="True" w30 {
        frame False {
        }
        frame True {
          n39 = local read "ENABLE INTERNAL MODULATION"() -> (w51:bool)
          n40 = local read "TRACK DATA PARAMETERS"() -> (w50:cluster{"MAIN FOLDER":path})
          n41 = Unbundle By Name(w50) -> ("MAIN FOLDER"=w49:path)
          n42 = case shown="True" w51 {
            frame False {
            }
            frame True {
              w54 = u16 1 items=["Channel 1"=1, "Channel 2"=2] ("Channel (1|2)")
              n43 = local read "NETWORK PARAMETERS"() -> (w53:cluster{"RP-IP 1":string, "RP-IP 2":string})
              n44 = Unbundle By Name(w53) -> ("RP-IP 2"=w52:string)
              n45 = call "RP-GEN SINUS-OUT.vi"("Amplitude(1V)"="Amplitude(1V)", "Frequency (Hz)"=10000000, "Channel (1|2)"=w54, "IP address"=w52) -> ()  [unwired: 1 out]
            }
          }
          n46 = Build Path(base path=w49, name or relative path=path "VOA calibration/PUMP.txt") -> (appended path=w46:path)
          n47 = Build Path(base path=w49, name or relative path=path "VOA calibration/PROBE.txt") -> (appended path=w45:path)
          n48 = local read "VOA Calibration cluster"() -> (w48:cluster{"PUMP":dbl[], "PROBE":dbl[]})
          n49 = call "RP-VOA CALIBRATION FIT.vi"("file path"=w46) -> ("Calibration array"=w44:dbl[])  [unwired: 2 in, 1 out]
          n50 = call "RP-VOA CALIBRATION FIT.vi"("file path"=w45) -> ("Calibration array"=w43:dbl[])  [unwired: 2 in, 1 out]
          n51 = Bundle By Name(cluster=w48, "PUMP"=w44, "PROBE"=w43) -> (w47:cluster{"PUMP":dbl[], "PROBE":dbl[]})
          n52 = local write "VOA Calibration cluster"(w47) -> ()
        }
      }
    }
    frame #3 {
      w70 = ""  # données (peuvent avoir n'importe quel type)
      # "attente libération des deux piles avant fermeture"
      # "MAIN"
      n53 = local read "NETWORK PARAMETERS"() -> (w59:cluster{"RP-IP 1":string, "RP-IP 2":string})
      n54 = local read "RP VNA SETTING"() -> (w66:T1)
      n55 = Unbundle By Name(w59) -> ("RP-IP 1"=w58:string)
      n56 = call "VNARP-Connexion.vi"("IP RP"=w58) -> ("sortie d'erreur"=w68:errorcluster, "ID de connexion"=w67:refnum<k5>)  [unwired: 1 in]
      n57 = Obtain Queue(element data type=w70) -> (queue out=w69:refnum<queue>, error out=w72:errorcluster)  [unwired: 4 in, 1 out]
      n58 = call "VNARP-SettingsUpdate.vi"("Error IN"=w68, "RP VNA SETTINGS IN"=w66, "ID de connexion IN"=w67) -> ("Error OUT"=w63:errorcluster, "Freq table"=w64:dbl[], "ID de connexion OUT"=w65:refnum<k5>)
      n59 = while {
        shift-right: [w536] -> w71
        shift-left: w72 -> [w538]
        tunnel: w69 -> [w539]
        tunnel: [w534] -> w62
        stop <- w534 stop-if-true
        n60 = event shown="[22] \"BTN RUN TRACK\": Mouse Up" {
          selector: _ -> [_ _ _ _ _ _ _ _ _ _ _ _ _ _ _ _ _ _ _ _ _ _ _ _]
          dyn-events: _ -> [_ _ _ _ _ _ _ _ _ _ _ _ _ _ _ _ _ _ _ _ _ _ _ _]
          timeout: 250 -> [_ _ _ _ _ _ _ _ _ _ _ _ _ _ _ _ _ _ _ _ _ _ _ _]
          tunnel: w539 -> [w544 _ w551 w555 _ _ w572 _ w597 w619 w645 w671 w694 w706 w735 _ _ _ _ _ w748 _ w774 _]
          tunnel: w538 -> [w542 _ w550 w554 _ _ w571 _ w596 w618 w644 w673 w693 w705 w734 _ _ _ _ _ w747 _ w775 _]
          tunnel: [w541 _ w549 w553 _ _ w570 _ w595 w617 w642 w672 w692 w704 w736 _ _ _ _ _ w746 _ w773 _] -> w536
          tunnel: [_ _ _ _ _ _ _ _ _ _ _ _ _ _ w732 _ _ _ _ _ _ _ _ _] -> w537
          event "BTN LOOP VNA": Value Change {
            n61 = event-data() -> ("NewVal"=w540:bool)  [unwired: 1 in]
            n62 = local write "LOOP ACT"(w540) -> ()
            n63 = Enqueue Element(queue=w544, element="VNA LOOP", error in (no error)=w542) -> (error out=w541:errorcluster)  [unwired: 1 in, 2 out]
          }
          event "BTN SAVE VNA STG TO TRACK": Value Change {
            n64 = event-data() -> ()  [unwired: 1 in, 1 out]
            n65 = local read "CHANNELS PARAMETERS"() -> (w548:T4)
            n66 = local read "VNA Settings cluster"() -> (w545:T9)
            n67 = local read "CHANNEL CHOICE VNA"() -> (w546:T3)
            n68 = Replace Array Subset(array=w548, new element=w545, index=w546) -> (w547:T4)
            n69 = local write "CHANNELS PARAMETERS"(w547) -> ()
          }
          event "BTN RUN VNA": Mouse Up {
            n70 = event-data() -> ()  [unwired: 1 in, 2 out]
            n71 = Enqueue Element(queue=w551, element="RUN VNA", error in (no error)=w550) -> (error out=w549:errorcluster)  [unwired: 1 in, 2 out]
          }
          event "PUMP", "PROBE": Mouse Up {
            n72 = event-data() -> ()  [unwired: 1 in, 2 out]
            n73 = Enqueue Element(queue=w555, element="POWER UPDATE", error in (no error)=w554) -> (error out=w553:errorcluster)  [unwired: 1 in, 2 out]
          }
          event "Hide/Show track data channel": Value Change {
            # "TO TEST ON ALPHA"
            n74 = event-data() -> ()  [unwired: 1 in, 2 out]
            n75 = local read "Hide/Show track data channel"() -> (w557:bool[])
            n76 = for {
              tunnel: w557 -> [w558] mode=indexing
              i -> [w559]
              n77 = flat-sequence {
                tunnel: w559 -> [w560]
                tunnel: w558 -> [w561]
                frame #0 {
                  n78 = property on="LIVE TRACK" class="WFGraph (strict)"("Active Plot"=w560) -> ()  [unwired: 2 in, 2 out]
                }
                frame #1 {
                  n79 = property on="LIVE TRACK" class="WFGraph (strict)"("Plot.Visible?"=w561) -> ()  [unwired: 2 in, 2 out]
                }
              }
            }
          }
          event "MAGNITUDE/PHASE": Value Change {
            n80 = event-data() -> ()  [unwired: 1 in, 2 out]
            n81 = flat-sequence {
              frame #0 {
                n82 = property on="MAGNITUDE/PHASE" class="XYGraph (strict)"("ActYScl"=0 ("Active Y Scale")) -> ()  [unwired: 2 in, 2 out]
              }
              frame #1 {
                n83 = local read "VNA DATA CLUSTER"() -> (w566:T7)
                n84 = Unbundle By Name(w566) -> ("MAGNITUDE TABLE"=w567:ext[])
                n85 = Array Max & Min(array=w567) -> (max value=w568:ext)  [unwired: 3 out]
                n86 = Multiply(x=1.1, y=w568) -> (x*y=w564:ext)
                n87 = property on="MAGNITUDE/PHASE" class="XYGraph (strict)"("YScale.Maximum"=w564, "YScale.Minimum"=0.0) -> ()  [unwired: 2 in, 2 out]
              }
            }
          }
          event "CHANNEL CHOICE VNA": Value Change {
            n88 = event-data() -> ()  [unwired: 1 in, 2 out]
            n89 = Enqueue Element(queue=w572, element="CHANNEL CHANGE", error in (no error)=w571) -> (error out=w570:errorcluster)  [unwired: 1 in, 2 out]
            n90 = One Button Dialog(message="TRIGGERED !") -> ()  [unwired: 1 in, 1 out]
          }
          event "BTN NEW TRACK": Mouse Up {
            n91 = event-data() -> ()  [unwired: 1 in, 2 out]
            n92 = Two Button Dialog(message="Initiate a new tracking session ?") -> (T button?=w574:bool)  [unwired: 2 in]
            n93 = case shown="True" w574 {
              frame False {
              }
              frame True {
                n94 = stacked-sequence {
                  frame #0 {
                    # "LOCK ALL CONTROLS"
                  }
                  frame #1 {
                    n95 = local read "TRACK DATA PARAMETERS"() -> (w580:cluster{"MAIN FOLDER":path})
                    n96 = local read "CHANNELS PARAMETERS"() -> (w582:T4)
                    n97 = local read "ASSAY NAME"() -> (w581:string)
                    n98 = Unbundle By Name(w580) -> ("MAIN FOLDER"=w579:path)
                    n99 = call "RP-TRACKDataStructBuild.vi"("CHANNELS PARAMETERS"=w582, "Track session name"=w581, "SensWay track data path"=w579) -> ("TRACK REPOSITERY"=w578:path, "Track File List"=w577:path[], "Track Repositery List"=w576:path[])
                    n100 = local write "Track Repositery List"(w576) -> ()
                    n101 = local write "TRACK REPOSITERY"(w578) -> ()
                    n102 = local write "Track File List"(w577) -> ()
                  }
                  frame #2 {
                    n103 = local read "CHANNELS PARAMETERS"() -> (w584:T4)
                    n104 = for {
                      tunnel: w584 -> [w594] mode=indexing
                      border: cluster{"CHANNEL":dbl, "KPI 1 TRACK":ext[]}[] [] -> [_]
                      i -> [w590]
                      n105 = Unbundle By Name(w594) -> ("CHANNEL TRACK ?"=w585:bool)
                      n106 = Select(t=dbl[] [0.0], s=w585, f=dbl[] []) -> (s? t:f=w588:dbl[])
                      n107 = Bundle By Name(cluster=cluster{"CHANNEL":dbl, "KPI 1 TRACK":ext[]} {"CHANNEL"=0.0, "KPI 1 TRACK"=[0.0]} ("TRACK DATA CLUSTER"), "CHANNEL"=w590, "KPI 1 TRACK"=w588) -> (w589:cluster{"CHANNEL":dbl, "KPI 1 TRACK":ext[]})
                      n108 = feedback #1() -> (w592:cluster{"CHANNEL":dbl, "KPI 1 TRACK":ext[]}[])
                      n109 = Build Array (concatenate)(w592, w589) -> (w593:cluster{"CHANNEL":dbl, "KPI 1 TRACK":ext[]}[])
                      n110 = feedback-in #1(w593) -> ()
                      n111 = local write "TRACK DATA CLUSTER TBL"(w593) -> ()
                    }
                  }
                  frame #3 {
                  }
                }
              }
            }
          }
          event "START", "STOP": Value Change {
            n112 = event-data() -> ()  [unwired: 1 in, 1 out]
            n113 = stacked-sequence {
              frame #0 {
                n114 = local read "STOP"() -> (w603:dbl)
                n115 = local read "START"() -> (w602:dbl)
                n116 = Subtract(x=w603, y=w602) -> (x-y=w604:dbl)
                n117 = Add(x=w603, y=w602) -> (x+y=w601:dbl)
                n118 = local write "SPAN"(w604) -> ()
                n119 = Divide(x=w601, y=2.0) -> (x/y=w599:dbl)
                n120 = local write "CENTER"(w599) -> ()
              }
              frame #1 {
                n121 = local read "Points N°"() -> (w609:i32)
                n122 = local read "SPAN"() -> (w608:dbl)
                n123 = Divide(x=w608, y=w609) -> (x/y=w607:dbl)
                n124 = Multiply(x=w607, y=1000.0) -> (x*y=w606:dbl)
                n125 = local write "SPACING"(w606) -> ()
              }
              frame #2 {
                w610 = 1000
                n126 = local read "START"() -> (w614:dbl)
                n127 = local read "STOP"() -> (w612:dbl)
                n128 = Multiply(x=w614, y=w610) -> (x*y=w613:dbl)
                n129 = Multiply(x=w610, y=w612) -> (x*y=w611:dbl)
                n130 = local read "RP VNA SETTING"() -> (w616:T1)
                n131 = Bundle By Name(cluster=w616, "F start"=w613, "F stop"=w611) -> (w615:T1)
                n132 = local write "RP VNA SETTING"(w615) -> ()
              }
            }
            n133 = Enqueue Element(queue=w597, element="UPDATE", error in (no error)=w596) -> (error out=w595:errorcluster)  [unwired: 1 in, 2 out]
          }
          event "CENTER", "SPAN": Value Change {
            n134 = event-data() -> ()  [unwired: 1 in, 1 out]
            n135 = stacked-sequence {
              frame #0 {
                w622 = 100.0 ("y")
                n136 = local read "CENTER"() -> (w626:dbl)
                n137 = local read "SPAN"() -> (w628:dbl)
                n138 = Divide(x=w628, y=2.0) -> (x/y=w625:dbl)
                n139 = Subtract(x=w626, y=w625) -> (x-y=w623:dbl)
                n140 = Add(x=w626, y=w625) -> (x+y=w629:dbl)
                n141 = local write "STOP"(w629) -> ()
                n142 = Greater Or Equal?(x=w623, y=w622) -> (x >= y?=w624:bool)
                n143 = Select(t=w623, s=w624, f=w622) -> (s? t:f=w621:dbl)
                n144 = local write "START"(w621) -> ()
              }
              frame #1 {
                n145 = local read "Points N°"() -> (w634:i32)
                n146 = local read "SPAN"() -> (w633:dbl)
                n147 = Divide(x=w633, y=w634) -> (x/y=w632:dbl)
                n148 = Multiply(x=w632, y=1000.0) -> (x*y=w631:dbl)
                n149 = local write "SPACING"(w631) -> ()
              }
              frame #2 {
                w635 = 1000
                n150 = local read "START"() -> (w639:dbl)
                n151 = local read "STOP"() -> (w637:dbl)
                n152 = Multiply(x=w639, y=w635) -> (x*y=w638:dbl)
                n153 = Multiply(x=w635, y=w637) -> (x*y=w636:dbl)
                n154 = local read "RP VNA SETTING"() -> (w641:T1)
                n155 = Bundle By Name(cluster=w641, "F start"=w638, "F stop"=w636) -> (w640:T1)
                n156 = local write "RP VNA SETTING"(w640) -> ()
              }
            }
            n157 = Enqueue Element(queue=w619, element="UPDATE", error in (no error)=w618) -> (error out=w617:errorcluster)  [unwired: 1 in, 2 out]
          }
          event "BTN ZOOM+": Mouse Up; "BTN ZOOM+": Value Change {
            n158 = event-data() -> ()  [unwired: 1 in, 1 out]
            n159 = stacked-sequence {
              frame #0 {
                n160 = local read "SPAN"() -> (w648:dbl)
                n161 = Multiply(x=w648, y=0.8) -> (x*y=w646:dbl)
                n162 = local write "SPAN"(w646) -> ()
              }
              frame #1 {
                n163 = local read "Points N°"() -> (w653:i32)
                n164 = local read "SPAN"() -> (w652:dbl)
                n165 = Divide(x=w652, y=w653) -> (x/y=w651:dbl)
                n166 = Multiply(x=w651, y=1000.0) -> (x*y=w650:dbl)
                n167 = local write "SPACING"(w650) -> ()
              }
              frame #2 {
                w655 = 100.0 ("y")
                n168 = local read "SPAN"() -> (w658:dbl)
                n169 = local read "CENTER"() -> (w660:dbl)
                n170 = Divide(x=w658, y=2.0) -> (x/y=w659:dbl)
                n171 = Subtract(x=w660, y=w659) -> (x-y=w656:dbl)
                n172 = Add(x=w660, y=w659) -> (x+y=w662:dbl)
                n173 = local write "STOP"(w662) -> ()
                n174 = Greater Or Equal?(x=w656, y=w655) -> (x >= y?=w657:bool)
                n175 = Select(t=w656, s=w657, f=w655) -> (s? t:f=w654:dbl)
                n176 = local write "START"(w654) -> ()
              }
              frame #3 {
                w663 = 1000
                n177 = local read "START"() -> (w667:dbl)
                n178 = local read "STOP"() -> (w665:dbl)
                n179 = Multiply(x=w667, y=w663) -> (x*y=w666:dbl)
                n180 = Multiply(x=w663, y=w665) -> (x*y=w664:dbl)
                n181 = local read "RP VNA SETTING"() -> (w669:T1)
                n182 = Bundle By Name(cluster=w669, "F start"=w666, "F stop"=w664) -> (w668:T1)
                n183 = local write "RP VNA SETTING"(w668) -> ()
              }
            }
            n184 = Enqueue Element(queue=w645, element="UPDATE", error in (no error)=w644) -> (error out=w642:errorcluster)  [unwired: 1 in, 2 out]
          }
          event "BTN RESET VNA": Mouse Up {
            n185 = event-data() -> ()  [unwired: 1 in, 1 out]
            n186 = flat-sequence {
              tunnel: w671 -> [w675]
              tunnel: [w675] -> w670
              frame #0 {
                w684 = u32 1000 ("Decimation")
                w682 = u32 2000000 ("Decimation")
                w683 = u32 200000 ("Decimation")
                w677 = u32 32700 ("F_corr")
                n187 = local read "RP VNA SETTING"() -> (w687:T1)
                n188 = local read "Points N°"() -> (w685:i32)
                n189 = Bundle By Name(cluster=w687, "F start"=w683, "F stop"=w682, "Sweep size"=w685, "Decimation"=u32 5000, "F_corr"=u32 0, "Ph_OUT1"=u32 0, "Ph_OUT2"=u32 0 ("F_corr"), "OUT_Lvl1"=w677, "OUT_Lvl2"=w677, "GPIO"=u32 0 ("F_corr")) -> (w686:T1)
                n190 = local write "RP VNA SETTING"(w686) -> ()
                n191 = Divide(x=w682, y=w684) -> (x/y=w688:dbl)
                n192 = Divide(x=w683, y=w684) -> (x/y=w689:dbl)
                n193 = local write "CENTER"(1050.0 ("Center")) -> ()
                n194 = local write "SPAN"(1900.0 ("Center")) -> ()
                n195 = local write "START"(w689) -> ()
                n196 = local write "STOP"(w688) -> ()
              }
            }
            n197 = Enqueue Element(queue=w670, element="UPDATE", error in (no error)=w673) -> (error out=w672:errorcluster)  [unwired: 1 in, 2 out]
          }
          event "Points N°": Value Change {
            n198 = event-data() -> ()  [unwired: 1 in, 1 out]
            n199 = stacked-sequence {
              frame #0 {
                n200 = local read "Points N°"() -> (w700:i32)
                n201 = local read "SPAN"() -> (w699:dbl)
                n202 = Divide(x=w699, y=w700) -> (x/y=w698:dbl)
                n203 = Multiply(x=w698, y=1000.0) -> (x*y=w697:dbl)
                n204 = local write "SPACING"(w697) -> ()
              }
              frame #1 {
                n205 = local read "RP VNA SETTING"() -> (w703:T1)
                n206 = local read "Points N°"() -> (w701:i32)
                n207 = Bundle By Name(cluster=w703, "Sweep size"=w701) -> (w702:T1)
                n208 = local write "RP VNA SETTING"(w702) -> ()
              }
            }
            n209 = Enqueue Element(queue=w694, element="UPDATE", error in (no error)=w693) -> (error out=w692:errorcluster)  [unwired: 1 in, 2 out]
          }
          event "BTN ZOOM-": Mouse Up {
            n210 = event-data() -> ()  [unwired: 1 in, 1 out]
            n211 = stacked-sequence {
              frame #0 {
                n212 = local read "SPAN"() -> (w710:dbl)
                n213 = Multiply(x=w710, y=1.2) -> (x*y=w708:dbl)
                n214 = local write "SPAN"(w708) -> ()
              }
              frame #1 {
                n215 = local read "Points N°"() -> (w715:i32)
                n216 = local read "SPAN"() -> (w714:dbl)
                n217 = Divide(x=w714, y=w715) -> (x/y=w713:dbl)
                n218 = Multiply(x=w713, y=1000.0) -> (x*y=w712:dbl)
                n219 = local write "SPACING"(w712) -> ()
              }
              frame #2 {
                w718 = 100.0 ("y")
                n220 = local read "SPAN"() -> (w720:dbl)
                n221 = local read "CENTER"() -> (w723:dbl)
                n222 = Divide(x=w720, y=2.0) -> (x/y=w722:dbl)
                n223 = Subtract(x=w723, y=w722) -> (x-y=w716:dbl)
                n224 = Add(x=w723, y=w722) -> (x+y=w724:dbl)
                n225 = Greater Or Equal?(x=w716, y=w718) -> (x >= y?=w719:bool)
                n226 = Select(t=w716, s=w719, f=w718) -> (s? t:f=w717:dbl)
                n227 = local write "STOP"(w724) -> ()
                n228 = local write "START"(w717) -> ()
              }
              frame #3 {
                w725 = 1000
                n229 = local read "START"() -> (w729:dbl)
                n230 = local read "STOP"() -> (w727:dbl)
                n231 = Multiply(x=w729, y=w725) -> (x*y=w728:dbl)
                n232 = Multiply(x=w725, y=w727) -> (x*y=w726:dbl)
                n233 = local read "RP VNA SETTING"() -> (w731:T1)
                n234 = Bundle By Name(cluster=w731, "F start"=w728, "F stop"=w726) -> (w730:T1)
                n235 = local write "RP VNA SETTING"(w730) -> ()
              }
            }
            n236 = Enqueue Element(queue=w706, element="UPDATE", error in (no error)=w705) -> (error out=w704:errorcluster)  [unwired: 1 in, 2 out]
          }
          event "BTN STOP": Value Change {
            n237 = event-data() -> ()  [unwired: 1 in, 1 out]
            n238 = Two Button Dialog(message="Are you sure you want to exit ?") -> (T button?=w732:bool)  [unwired: 2 in]
            n239 = case shown="True" w732 {
              tunnel: [w737 w740] -> w736
              tunnel: w735 -> [_ w739]
              tunnel: w734 -> [w737 w738]
              frame False {
              }
              frame True {
                n240 = Enqueue Element(queue=w739, element="STOP", error in (no error)=w738) -> (error out=w740:errorcluster)  [unwired: 1 in, 2 out]
              }
            }
          }
          event "PANEL GENERAL SETTINGS": Value Change {
            n241 = event-data() -> ()  [unwired: 1 in, 2 out]
            n242 = local write "MAIN TAB"(enum32{"Page 1", "Page 4", "Page 2", "Page 3"}."Page 3" ("Tab Control")) -> ()
          }
          event Timeout {
            n243 = event-data() -> ()  [unwired: 1 in, 2 out]
          }
          event "PANEL TRACK SETTINGS": Value Change {
            n244 = event-data() -> ()  [unwired: 1 in, 2 out]
            n245 = local write "MAIN TAB"(enum32{"Page 1", "Page 4", "Page 2", "Page 3"}."Page 2" ("Tab Control")) -> ()
          }
          event "PANEL VNA": Value Change {
            n246 = event-data() -> ()  [unwired: 1 in, 2 out]
            n247 = local write "MAIN TAB"(enum32{"Page 1", "Page 4", "Page 2", "Page 3"}."Page 1" ("Tab Control")) -> ()
          }
          event "PANEL TRACKING": Value Change {
            n248 = event-data() -> ()  [unwired: 1 in, 2 out]
            n249 = local write "MAIN TAB"(enum32{"Page 1", "Page 4", "Page 2", "Page 3"}."Page 4" ("Tab Control")) -> ()
          }
          event "BTN Center to max": Mouse Up; "BTN Center to max": Value Change {
            n250 = event-data() -> ()  [unwired: 1 in, 2 out]
            n251 = stacked-sequence {
              frame #0 {
                # "ATTENTION ! CONFUSION  freq table"
                n252 = local read "VNA DATA CLUSTER"() -> (w753:T7)
                n253 = Unbundle By Name(w753) -> ("FREQUENCY TABLE"=w752:ext[], "MAGNITUDE TABLE"=w751:ext[])
                n254 = Array Max & Min(array=w751) -> (max index (indices)=w756:i32)  [unwired: 3 out]
                n255 = Index Array(array=w752, index=w756) -> (element=w755:ext)
                n256 = Divide(x=w755, y=1000.0) -> (x/y=w750:ext)
                n257 = local write "CENTER"(w750) -> ()
                n258 = property on="CENTER" class="DigNum (strict)"("Val(Sgnl)"=w750) -> ()  [unwired: 2 in, 2 out]
              }
              frame #1 {
                w759 = 1000
                n259 = local read "START"() -> (w757:dbl)
                n260 = local read "STOP"() -> (w758:dbl)
                n261 = Multiply(x=w757, y=w759) -> (x*y=w761:dbl)
                n262 = Multiply(x=w759, y=w758) -> (x*y=w760:dbl)
                n263 = local read "RP VNA SETTING"() -> (w763:T1)
                n264 = Bundle By Name(cluster=w763, "F start"=w761, "F stop"=w760) -> (w762:T1)
                n265 = local write "RP VNA SETTING"(w762) -> ()
              }
            }
            n266 = Enqueue Element(queue=w748, element="UPDATE", error in (no error)=w747) -> (error out=w746:errorcluster)  [unwired: 1 in, 2 out]
          }
          event "BTN AF VNA": Mouse Up {
            n267 = event-data() -> ()  [unwired: 1 in, 2 out]
            n268 = local read "AUTOFOCUS PARAMETERS"() -> (w765:cluster{"ITERATIONS":i32})
            n269 = Unbundle By Name(w765) -> ("ITERATIONS"=w764:i32)
            n270 = for {
              N: w764 -> [_]
              tunnel: [w768] -> w766
              n271 = flat-sequence {
                tunnel: [w769] -> w768
                frame #0 {
                  w769 = FALSE ("Valeur (Signalisation)")
                  n272 = property on="BTN Center to max" class="Bool (strict)"("Val(Sgnl)"=w769) -> ()  [unwired: 2 in, 2 out]
                }
                frame #1 {
                  n273 = property on="BTN ZOOM+" class="Bool (strict)"("Val(Sgnl)"=FALSE ("Valeur (Signalisation)")) -> ()  [unwired: 2 in, 2 out]
                }
              }
              n274 = Wait (ms)(milliseconds to wait=u32 250 ("attente (ms)")) -> ()  [unwired: 1 out]
            }
            n275 = property on="BTN Center to max" class="Bool (strict)"("Val(Sgnl)"=w766) -> ()  [unwired: 2 in, 2 out]
          }
          event "BTN RUN TRACK": Mouse Up {
            w771 = TRUE ("x")
            n276 = event-data() -> ()  [unwired: 1 in, 2 out]
            n277 = local write "LOOP ACT"(w771) -> ()
            n278 = Not(x=w771) -> (.not. x?=w772:bool)
            n279 = property on="BTN PAUSE TRACK" class="Bool (strict)"("Visible"=w771) -> ()  [unwired: 2 in, 2 out]
            n280 = Enqueue Element(queue=w774, element="TRACK", error in (no error)=w775) -> (error out=w773:errorcluster)  [unwired: 1 in, 2 out]
            n281 = property on="BTN RUN TRACK" class="Bool (strict)"("Visible"=w772) -> ()  [unwired: 2 in, 2 out]
          }
          event "BTN PAUSE TRACK": Mouse Up {
            w777 = FALSE ("x")
            n282 = event-data() -> ()  [unwired: 1 in, 2 out]
            n283 = local write "LOOP ACT"(w777) -> ()
            n284 = Not(x=w777) -> (.not. x?=w778:bool)
            n285 = property on="BTN PAUSE TRACK" class="Bool (strict)"("Visible"=w777) -> ()  [unwired: 2 in, 2 out]
            n286 = property on="BTN RUN TRACK" class="Bool (strict)"("Visible"=w778) -> ()  [unwired: 2 in, 2 out]
          }
        }
        n287 = Or(x=w536, y=w537) -> (x .or. y?=w534:bool)
        n288 = Wait (ms)(milliseconds to wait=u32 50 ("attente (ms)")) -> ()  [unwired: 1 out]
      }
      n289 = while {
        tunnel: w69 -> [w81]
        tunnel: w65 -> [w79]
        tunnel: w64 -> [w78]
        tunnel: w63 -> [w77]
        tunnel: [w76] -> w61
        border: dbl[] [0.0] -> [_]
        stop <- w76 stop-if-true
        n290 = Dequeue Element(queue=w81) -> (queue out=w80:refnum<queue>, element=w82:string, error out=w83:errorcluster)  [unwired: 2 in, 1 out]
        n291 = case shown="No Error" w83 {
          selector: w83 -> [w88 _]
          tunnel: w82 -> [w90 _]
          tunnel: [w84 TRUE] -> w76
          tunnel: w80 -> [w89 _]
          tunnel: w79 -> [w87 _]
          tunnel: w78 -> [w86 _]
          tunnel: w77 -> [w85 _]
          frame No Error {
            n292 = case shown="\"UPDATE\"" w90 {
              selector: w90 -> [w97 w135 w197 w413 _ w478 w483 w503 w527]
              tunnel: w89 -> [w95 w130 w193 _ _ _ _ _ _]
              tunnel: w88 -> [_ _ _ _ _ _ _ _ _]
              tunnel: w87 -> [w94 w132 w195 w411 _ _ w482 _ w530]
              tunnel: w86 -> [w93 _ _ _ _ _ _ _ _]
              tunnel: w85 -> [w92 w131 w194 w410 _ _ w481 _ w529]
              tunnel: [FALSE FALSE FALSE FALSE FALSE FALSE FALSE FALSE TRUE] -> w84
              frame "VNA LOOP", Default {
                n293 = local write "STATUS"(w97) -> ()
                n294 = stacked-sequence {
                  tunnel: w94 -> [w107 _]
                  tunnel: w93 -> [_ _]
                  tunnel: w92 -> [w106 _]
                  tunnel: w95 -> [_ w126]
                  frame #0 {
                    (unwired) 10 ("kernel size (pts)")
                    n295 = local read "SPECTRUM POST PROCESSING PARAMETERS"() -> (w102:cluster{"N° SMOOTHING POINTS":i32})
                    n296 = local read "RP VNA SETTING"() -> (w120:T1)
                    n297 = Unbundle By Name(w102) -> ("N° SMOOTHING POINTS"=w101:i32)
                    n298 = Unbundle By Name(w120) -> ("Sweep size"=w119:u32)
                    n299 = local read "RAW Freq table"() -> (w115:dbl[])
                    n300 = local read "VNA DATA CLUSTER"() -> (w105:T7)
                    n301 = call "VNARP-CASES.vi"("entrée d'erreur (pas d'erreur)"=w106, "Setting"=u32 0, "Énum"=T10."SWEEP START", "ID de connexion"=w107) -> ("sortie d'erreur"=w116:errorcluster, "ID de connexion en sortie"=w121:refnum<k5>)  [unwired: 3 in]
                    n302 = call "VNARP-Read.vi"("ID de connexion"=w121, "entrée d'erreur (pas d'erreur)"=w116, "SIZE"=w119) -> ("MAGNITUDE 1"=w118:sgl[], "PHASE 1"=w117:dbl[])  [unwired: 9 in, 6 out]
                    n303 = call "VNARP-BOXCAR.vi"("Y IN"=w118, "kernel size (pts)"=w101, "Freq table IN"=w115) -> ("Y OUT"=w99:dbl[], "Freq table OUT"=w114:dbl[])  [unwired: 1 in]
                    n304 = call "VNARP-BOXCAR.vi"("Y IN"=w117, "kernel size (pts)"=w101, "Freq table IN"=w115) -> ("Y OUT"=w98:dbl[], "Freq table OUT"=w103:dbl[])  [unwired: 1 in]
                    n305 = Bundle By Name(cluster=w105, "FREQUENCY TABLE"=w103, "MAGNITUDE TABLE"=w99, "PHASE TABLE"=w98) -> (w104:T7)
                    n306 = Build Cluster Array(w114, w99) -> (w112:cluster{dbl, dbl}[])
                    n307 = Build Cluster Array(w103, w98) -> (w113:cluster{dbl, dbl}[])
                    n308 = local write "VNA DATA CLUSTER"(w104) -> ()
                    n309 = Bundle(w112) -> (w111:cluster{cluster{dbl, dbl}[]})  [unwired: 1 in]
                    n310 = Bundle(w113) -> (w110:cluster{cluster{dbl, dbl}[]})  [unwired: 1 in]
                    n311 = Build Array(w111, w110) -> (w100:cluster{cluster{dbl, dbl}[]}[])
                    n312 = local write "MAGNITUDE/PHASE"(w100) -> ()
                    n313 = property on="MAGNITUDE/PHASE" class="XYGraph (strict)"("Val(Sgnl)"=w100) -> ()  [unwired: 2 in, 2 out]
                  }
                  frame #1 {
                    n314 = local read "LOOP ACT"() -> (w125:bool)
                    n315 = Select(t="VNA LOOP" ("element"), s=w125, f="WAIT" ("element")) -> (s? t:f=w124:string)
                    n316 = Enqueue Element(queue=w126, element=w124) -> ()  [unwired: 2 in, 3 out]
                    n317 = stacked-sequence {
                      frame #0 {
                        n318 = local write "ACQ Indicator"(TRUE ("ACQ Indicator")) -> ()
                      }
                      frame #1 {
                        n319 = Wait (ms)(milliseconds to wait=u32 100 ("attente (ms)")) -> ()  [unwired: 1 out]
                      }
                      frame #2 {
                        n320 = local write "ACQ Indicator"(FALSE ("ACQ Indicator")) -> ()
                      }
                    }
                  }
                }
                n321 = Wait (ms)(milliseconds to wait=u32 10 ("attente (ms)")) -> ()  [unwired: 1 out]
              }
              frame "TRACK OBS" {
                n322 = local write "STATUS"(w135) -> ()
                n323 = stacked-sequence {
                  tunnel: w132 -> [w145 _ _ _]
                  tunnel: w131 -> [w144 _ _ _]
                  tunnel: w130 -> [_ _ _ w192]
                  frame #0 {
                    n324 = local read "SPECTRUM POST PROCESSING PARAMETERS"() -> (w138:cluster{"N° SMOOTHING POINTS":i32})
                    n325 = local read "RP VNA SETTING"() -> (w158:T1)
                    n326 = Unbundle By Name(w138) -> ("N° SMOOTHING POINTS"=w137:i32)
                    n327 = Unbundle By Name(w158) -> ("Sweep size"=w157:u32)
                    n328 = local read "RAW Freq table"() -> (w153:dbl[])
                    n329 = call "VNARP-CASES.vi"("entrée d'erreur (pas d'erreur)"=w144, "Setting"=u32 0, "Énum"=T10."SWEEP START", "ID de connexion"=w145) -> ("sortie d'erreur"=w154:errorcluster, "ID de connexion en sortie"=w159:refnum<k5>)  [unwired: 3 in]
                    n330 = call "VNARP-Read.vi"("ID de connexion"=w159, "entrée d'erreur (pas d'erreur)"=w154, "SIZE"=w157) -> ("MAGNITUDE 1"=w156:sgl[], "PHASE 1"=w155:dbl[])  [unwired: 9 in, 6 out]
                    n331 = call "VNARP-BOXCAR.vi"("Y IN"=w156, "kernel size (pts)"=w137, "Freq table IN"=w153) -> ("Y OUT"=w140:dbl[], "Freq table OUT"=w152:dbl[])  [unwired: 1 in]
                    n332 = call "VNARP-BOXCAR.vi"("Y IN"=w155, "kernel size (pts)"=w137, "Freq table IN"=w153) -> ("Y OUT"=w139:dbl[], "Freq table OUT"=w141:dbl[])  [unwired: 1 in]
                    n333 = local read "VNA DATA CLUSTER"() -> (w143:T7)
                    n334 = Build Cluster Array(w152, w140) -> (w150:cluster{dbl, dbl}[])
                    n335 = Build Cluster Array(w141, w139) -> (w151:cluster{dbl, dbl}[])
                    n336 = Bundle By Name(cluster=w143, "FREQUENCY TABLE"=w141, "MAGNITUDE TABLE"=w140, "PHASE TABLE"=w139) -> (w142:T7)
                    n337 = Bundle(w150) -> (w149:cluster{cluster{dbl, dbl}[]})  [unwired: 1 in]
                    n338 = Bundle(w151) -> (w148:cluster{cluster{dbl, dbl}[]})  [unwired: 1 in]
                    n339 = Build Array(w149, w148) -> (w136:cluster{cluster{dbl, dbl}[]}[])
                    n340 = local write "MAGNITUDE/PHASE"(w136) -> ()
                    n341 = property on="MAGNITUDE/PHASE" class="XYGraph (strict)"("Val(Sgnl)"=w136) -> ()  [unwired: 2 in, 2 out]
                    n342 = local write "VNA DATA CLUSTER"(w142) -> ()
                  }
                  frame #1 {
                    n343 = local read "RP VNA SETTING"() -> (w169:T1)
                    n344 = local read "VNA DATA CLUSTER"() -> (w172:T7)
                    n345 = Unbundle By Name(w169) -> ("Sweep size"=w168:u32)
                    n346 = Max & Min(x=500 ("Fit length"), y=w168) -> (min(x,y)=w166:u32)  [unwired: 1 out]
                    n347 = Unbundle By Name(w172) -> ("FREQUENCY TABLE"=w165:ext[], "MAGNITUDE TABLE"=w164:ext[])
                    n348 = call "VNARP PARABOLA FIT.vi"("Freq Table IN"=w165, "Fit length"=w166, "Y IN"=w164) -> ("Parabol max position"=w171:dbl)  [unwired: 3 out]
                    n349 = feedback #2() -> (w170:dbl[])
                    n350 = Build Array (concatenate)(w170, w171) -> (w162:dbl[])
                    n351 = call "Search Unsorted 1D Array.vim"("element"=0.0, "unsorted 1D array"=w162) -> ("index of element"=w163:i32)  [unwired: 9 in]
                    n352 = Delete From Array(array=w162, index=w163) -> (array with subset deleted=w160:dbl[])  [unwired: 1 in, 1 out]
                    n353 = feedback-in #2(w160) -> ()
                    n354 = local write "track data"(w160) -> ()
                  }
                  frame #2 {
                    n355 = local read "TEMPORAL SMOOTHING"() -> (w175:i32)
                    n356 = local read "track data"() -> (w173:dbl[])
                    n357 = Array Size(array=w173) -> (size(s)=w177:i32)
                    n358 = Subtract(x=w177, y=w175) -> (x-y=w178:i32)
                    n359 = for {
                      N: w178 -> [_]
                      tunnel: w175 -> [w186]
                      tunnel: w173 -> [w187]
                      tunnel: [w183] -> w176 mode=indexing
                      i -> [w185]
                      n360 = Array Subset(array=w187, index=w185, length=w186) -> (w184:dbl[])
                      n361 = call-poly <vilib>:"Mean.vi"("X"=w184) -> ("mean"=w183:dbl)  [unwired: 1 out]
                    }
                    n362 = local read "N°POINTS TO DISPLAY"() -> (w179:i32)
                    n363 = Array Size(array=w176) -> (size(s)=w181:i32)
                    n364 = Subtract(x=w181, y=w179) -> (x-y=w180:i32)
                    n365 = Max & Min(x=0.0, y=w180) -> (max(x,y)=w182:dbl)  [unwired: 1 out]
                    n366 = Array Subset(array=w176, index=w182, length=w179) -> ()  [unwired: 1 out]
                  }
                  frame #3 {
                    n367 = local read "LOOP ACT"() -> (w191:bool)
                    n368 = Select(t="TRACK" ("element"), s=w191, f="WAIT" ("element")) -> (s? t:f=w190:string)
                    n369 = Enqueue Element(queue=w192, element=w190) -> ()  [unwired: 2 in, 3 out]
                  }
                }
                n370 = Wait (ms)(milliseconds to wait=u32 10 ("attente (ms)")) -> ()  [unwired: 1 out]
              }
              frame "TRACK" {
                n371 = local write "STATUS"(w197) -> ()
                n372 = stacked-sequence {
                  tunnel: w195 -> [_ w204 _]
                  tunnel: w194 -> [_ w203 _]
                  tunnel: w193 -> [_ w202 w405]
                  frame #0 {
                    n373 = local read "DELAY BETWEEN TRIG (s)"() -> (w200:i32)
                    n374 = Multiply(x=w200, y=u32 1000 ("attente (ms)")) -> (x*y=w199:u32)
                    n375 = Wait (ms)(milliseconds to wait=w199) -> ()  [unwired: 1 out]
                  }
                  frame #1 {
                    n376 = local read "CHANNELS PARAMETERS"() -> (w201:T4)
                    n377 = for {
                      tunnel: w201 -> [w210] mode=indexing
                      tunnel: w204 -> [w209]
                      tunnel: w203 -> [w208]
                      tunnel: w202 -> [w206]
                      tunnel: w201 -> [w205]
                      i -> [w207]
                      n378 = Unbundle By Name(w210) -> ("CHANNEL TRACK ?"=w211:bool)
                      n379 = case shown="True" w211 {
                        tunnel: w210 -> [_ w213]
                        tunnel: w209 -> [_ w214]
                        tunnel: w208 -> [_ w216]
                        tunnel: w207 -> [_ w215]
                        tunnel: w206 -> [_ _]
                        tunnel: w205 -> [_ w212]
                        frame False {
                        }
                        frame True {
                          n380 = stacked-sequence {
                            tunnel: w216 -> [_ w228 _ _ _ w257 w274 _ _ _ _ _ _ _]
                            tunnel: w215 -> [w217 _ _ _ w248 _ _ w296 w301 w317 _ _ _ _]
                            tunnel: w214 -> [_ w219 _ _ _ w254 w272 _ _ _ _ _ _ _]
                            tunnel: w213 -> [_ w218 _ _ w249 _ _ _ _ _ _ _ _ _]
                            tunnel: w212 -> [_ _ _ _ w247 _ _ _ _ _ _ _ _ _]
                            frame #0 {
                              # "ATTENTION : do not trig channel choice change event !!!!"
                              # "switch"
                              n381 = local write "CHANNELS IND TRACK"(w217) -> ()
                              n382 = local write "CHANNEL CHOICE VNA"(w217) -> ()
                            }
                            frame #1 {
                              n383 = local write "VNA Settings cluster"(w218) -> ()
                              n384 = local read "RP VNA SETTING"() -> (w231:T1)
                              n385 = call "VNARP-VNASETTING CLTR MANAGMENT.vi"("VNA Settings cluster"=w218, "RP VNA SETTING"=w231) -> ("OUTPUT VNA SETTINGS"=w229:T1)  [unwired: 1 in]
                              n386 = local write "RP VNA SETTING"(w229) -> ()
                              n387 = call "VNARP-SettingsUpdate.vi"("Error IN"=w228, "RP VNA SETTINGS IN"=w229, "ID de connexion IN"=w219) -> ("Freq table"=w230:dbl[])  [unwired: 2 out]
                              n388 = local write "RAW Freq table"(w230) -> ()
                              n389 = Unbundle By Name(w218) -> ("START 2"=w221:dbl, "STOP 2"=w227:dbl, "CENTER 2"=w226:dbl, "SPAN 2"=w225:dbl, "PUMP"=w220:dbl, "PROBE"=w224:dbl, "Points N° 2"=w223:i32, "SPACING 2"=w222:dbl)
                              n390 = local write "Points N°"(w223) -> ()
                              n391 = local write "SPACING"(w222) -> ()
                              n392 = local write "CENTER"(w226) -> ()
                              n393 = local write "START"(w221) -> ()
                              n394 = local write "STOP"(w227) -> ()
                              n395 = local write "PROBE"(w224) -> ()
                              n396 = local write "SPAN"(w225) -> ()
                              n397 = local write "PUMP"(w220) -> ()
                              n398 = property on="START" class="DigNum (strict)"("Val(Sgnl)"=w221) -> ()  [unwired: 2 in, 2 out]
                              n399 = property on="PUMP" class="Slide (strict)"("Val(Sgnl)"=w220) -> ()  [unwired: 2 in, 2 out]
                            }
                            frame #2 {
                              w240 = u16 0 items=["AOUT0", "AOUT1", "AOUT2", "AOUT3"] ("Pin #")
                              w239 = u16 1 items=["AOUT0", "AOUT1", "AOUT2", "AOUT3"] ("Pin #")
                              n400 = local read "VOA Calibration cluster"() -> (w238:cluster{"PUMP":dbl[], "PROBE":dbl[]})
                              n401 = local read "NETWORK PARAMETERS"() -> (w242:cluster{"RP-IP 1":string, "RP-IP 2":string})
                              n402 = Unbundle By Name(w242) -> ("RP-IP 2"=w241:string)
                              n403 = Unbundle By Name(w238) -> ("PUMP"=w233:dbl[], "PROBE"=w236:dbl[])
                              n404 = local read "PUMP"() -> (w234:dbl)
                              n405 = local read "PROBE"() -> (w237:dbl)
                              n406 = call "RP-VOA CONVERSION P to V.vi"("Calibration points"=w233, "% power"=w234) -> ("DAC Voltage"=w232:dbl)
                              n407 = call "RP-VOA CONVERSION P to V.vi"("Calibration points"=w236, "% power"=w237) -> ("DAC Voltage"=w235:dbl)
                              n408 = call "RP-ANALOG-OUT.vi"("Analog Voltage Value (V)"=w232, "Pin #"=w240, "IP address"=w241) -> ()  [unwired: 1 out]
                              n409 = call "RP-ANALOG-OUT.vi"("Analog Voltage Value (V)"=w235, "Pin #"=w239, "IP address"=w241) -> ()  [unwired: 1 out]
                            }
                            frame #3 {
                              n410 = local read "VNA Settings cluster"() -> (w246:T9)
                              n411 = local read "PROBE"() -> (w244:dbl)
                              n412 = local read "PUMP"() -> (w245:dbl)
                              n413 = Bundle By Name(cluster=w246, "PUMP"=w245, "PROBE"=w244) -> (w243:T9)
                              n414 = local write "VNA Settings cluster"(w243) -> ()
                            }
                            frame #4 {
                              n415 = local read "VNA Settings cluster"() -> (w252:T9)
                              n416 = Unbundle By Name(w249) -> ("CHANNEL TRACK ?"=w251:bool)
                              n417 = Bundle By Name(cluster=w252, "CHANNEL TRACK ?"=w251) -> (w250:T9)
                              n418 = Replace Array Subset(array=w247, new element=w250, index=w248) -> (w253:T4)
                              n419 = local write "CHANNELS PARAMETERS"(w253) -> ()
                            }
                            frame #5 {
                              # "wait for stab"
                              n420 = local read "DELAY AFTER SWITCH (s)"() -> (w256:i32)
                              n421 = Equal To 0?(x=w256) -> (x = 0?=w255:bool)
                              n422 = case shown="False" w255 {
                                tunnel: w257 -> [w259 _]
                                tunnel: w254 -> [w258 _]
                                frame False {
                                n423 = Tick Count (ms)() -> (millisecond timer value=w260:u32)
                                n424 = while {
                                tunnel: w260 -> [w269]
                                tunnel: w259 -> [w263]
                                tunnel: w258 -> [w262]
                                stop <- w264 stop-if-true
                                n425 = flat-sequence {
                                tunnel: w263 -> [_]
                                tunnel: w262 -> [_]
                                tunnel: [w270] -> w261
                                frame #0 {
                                }
                                frame #1 {
                                n426 = Tick Count (ms)() -> (millisecond timer value=w270:u32)
                                }
                                }
                                n427 = local read "DELAY AFTER SWITCH (s)"() -> (w268:i32)
                                n428 = Subtract(x=w261, y=w269) -> (x-y=w266:u32)
                                n429 = Multiply(x=w268, y=1000) -> (x*y=w265:i32)
                                n430 = Greater Or Equal?(x=w266, y=w265) -> (x >= y?=w264:bool)
                                }
                                }
                                frame True {
                                }
                              }
                            }
                            frame #6 {
                              # "AVERAGING IS MISSING !"
                              n431 = local read "SPECTRUM POST PROCESSING PARAMETERS"() -> (w278:cluster{"N° SMOOTHING POINTS":i32})
                              n432 = Unbundle By Name(w278) -> ("N° SMOOTHING POINTS"=w277:i32)
                              n433 = local read "RP VNA SETTING"() -> (w294:T1)
                              n434 = Unbundle By Name(w294) -> ("Sweep size"=w293:u32)
                              n435 = local read "RAW Freq table"() -> (w289:dbl[])
                              n436 = call "VNARP-CASES.vi"("entrée d'erreur (pas d'erreur)"=w274, "Setting"=u32 0, "Énum"=T10."SWEEP START", "ID de connexion"=w272) -> ("sortie d'erreur"=w290:errorcluster, "ID de connexion en sortie"=w295:refnum<k5>)  [unwired: 3 in]
                              n437 = local read "CHANNEL CHOICE VNA"() -> (w273:T3)
                              n438 = call "VNARP-Read.vi"("ID de connexion"=w295, "entrée d'erreur (pas d'erreur)"=w290, "SIZE"=w293) -> ("MAGNITUDE 1"=w292:sgl[], "PHASE 1"=w291:dbl[])  [unwired: 9 in, 6 out]
                              n439 = call "VNARP-BOXCAR.vi"("Y IN"=w292, "kernel size (pts)"=w277, "Freq table IN"=w289) -> ("Y OUT"=w280:dbl[], "Freq table OUT"=w288:dbl[])  [unwired: 1 in]
                              n440 = call "VNARP-BOXCAR.vi"("Y IN"=w291, "kernel size (pts)"=w277, "Freq table IN"=w289) -> ("Y OUT"=w279:dbl[], "Freq table OUT"=w281:dbl[])  [unwired: 1 in]
                              n441 = Build Cluster Array(w288, w280) -> (w286:cluster{dbl, dbl}[])
                              n442 = Build Cluster Array(w281, w279) -> (w287:cluster{dbl, dbl}[])
                              n443 = local read "VNA DATA CLUSTER"() -> (w283:T7)
                              n444 = Bundle By Name(cluster=w283, "CHANNEL"=w273, "FREQUENCY TABLE"=w281, "MAGNITUDE TABLE"=w280, "PHASE TABLE"=w279) -> (w282:T7)
                              n445 = Bundle(w286) -> (w285:cluster{cluster{dbl, dbl}[]})  [unwired: 1 in]
                              n446 = Bundle(w287) -> (w284:cluster{cluster{dbl, dbl}[]})  [unwired: 1 in]
                              n447 = Build Array(w285, w284) -> (w271:cluster{cluster{dbl, dbl}[]}[])
                              n448 = local write "MAGNITUDE/PHASE"(w271) -> ()
                              n449 = property on="MAGNITUDE/PHASE" class="XYGraph (strict)"("Val(Sgnl)"=w271) -> ()  [unwired: 2 in, 2 out]
                              n450 = local write "VNA DATA CLUSTER"(w282) -> ()
                            }
                            frame #7 {
                              n451 = local read "VNA DATA CLUSTER TBL"() -> (w298:T8)
                              n452 = local read "VNA DATA CLUSTER"() -> (w297:T7)
                              n453 = Replace Array Subset(array=w298, new element=w297, index=w296) -> (w299:T8)
                              n454 = local write "VNA DATA CLUSTER TBL"(w299) -> ()
                            }
                            frame #8 {
                              n455 = local read "BTN AUTOSAVE RAW DATA"() -> (w300:bool)
                              n456 = case shown="True" w300 {
                                tunnel: w301 -> [_ w303]
                                frame False {
                                }
                                frame True {
                                # "save to file vna"
                                n457 = local read "VNA DATA CLUSTER TBL"() -> (w314:T8)
                                n458 = local read "Track Repositery List"() -> (w304:path[])
                                n459 = Tick Count (ms)() -> (millisecond timer value=w312:u32)
                                n460 = Number To Decimal String(number=w312) -> (decimal integer string=w311:string)  [unwired: 1 in]
                                n461 = call "RP-VNA DATA TBL Extract.vi"("VNA DATA CLUSTER TBL"=w314, "index"=w303) -> ("appended array"=w313:ext[][])  [unwired: 2 in, 1 out]
                                n462 = Concatenate Strings("RAW VNA DATA " ("string"), w311, ".txt" ("string")) -> (w309:string)
                                n463 = Index Array(array=w304, index=w303) -> (element=w302:path)
                                n464 = Build Path(base path=w302, name or relative path=w309) -> (appended path=w308:path)
                                n465 = call-poly <vilib>:"Write Delimited Spreadsheet.vi"("file path (dialog if empty)"=w308, "format (%.3f)"="%.6f", "2D data"=w313, "transpose? (no:F)"=TRUE) -> ()  [unwired: 10 in, 2 out]
                                }
                              }
                            }
                            frame #9 {
                              # "add to track kpi tables"
                              n466 = local read "TRACK DATA CLUSTER TBL"() -> (w318:cluster{"CHANNEL":dbl, "KPI 1 TRACK":ext[]}[])
                              n467 = local read "VNA DATA CLUSTER"() -> (w329:T7)
                              n468 = local read "RP VNA SETTING"() -> (w328:T1)
                              n469 = Unbundle By Name(w328) -> ("Sweep size"=w327:u32)
                              n470 = Unbundle By Name(w329) -> ("FREQUENCY TABLE"=w325:ext[], "MAGNITUDE TABLE"=w324:ext[])
                              n471 = Index Array(array=w318, index=w317) -> (element=w320:cluster{"CHANNEL":dbl, "KPI 1 TRACK":ext[]})
                              n472 = Unbundle By Name(w320) -> ("KPI 1 TRACK"=w322:ext[])
                              n473 = Max & Min(x=500 ("Fit length"), y=w327) -> (min(x,y)=w326:u32)  [unwired: 1 out]
                              n474 = call "VNARP PARABOLA FIT.vi"("Freq Table IN"=w325, "Fit length"=w326, "Y IN"=w324) -> ("Parabol max position"=w315:dbl)  [unwired: 3 out]
                              n475 = Build Array (concatenate)(w322, w315) -> (w321:ext[])
                              n476 = Bundle By Name(cluster=w320, "CHANNEL"=w317, "KPI 1 TRACK"=w321) -> (w319:cluster{"CHANNEL":dbl, "KPI 1 TRACK":ext[]})
                              n477 = Replace Array Subset(array=w318, new element=w319, index=w317) -> (w316:cluster{"CHANNEL":dbl, "KPI 1 TRACK":ext[]}[])
                              n478 = local write "TRACK DATA CLUSTER TBL"(w316) -> ()
                            }
                            frame #10 {
                              n479 = local read "TRACK DATA CLUSTER TBL"() -> (w333:cluster{"CHANNEL":dbl, "KPI 1 TRACK":ext[]}[])
                              n480 = for {
                                tunnel: w333 -> [w358] mode=indexing
                                tunnel: [w336] -> w332 mode=indexing
                                tunnel: [w335] -> w331 mode=indexing
                                tunnel: [w334] -> w330 mode=indexing
                                n481 = local read "TEMPORAL SMOOTHING"() -> (w355:i32)
                                n482 = Unbundle By Name(w358) -> ("KPI 1 TRACK"=w354:ext[])
                                n483 = Array Size(array=w354) -> (size(s)=w356:i32)
                                n484 = Subtract(x=w356, y=w355) -> (x-y=w357:i32)
                                n485 = for {
                                N: w357 -> [_]
                                tunnel: w355 -> [w362]
                                tunnel: w354 -> [w363]
                                tunnel: [w359] -> w343 mode=indexing
                                i -> [w361]
                                n486 = Array Subset(array=w363, index=w361, length=w362) -> (w360:ext[])
                                n487 = call-poly <vilib>:"Mean.vi"("X"=w360) -> ("mean"=w359:dbl)  [unwired: 1 out]
                                }
                                n488 = Delete From Array(array=w343, length=1, index=0) -> (array with subset deleted=w335:dbl[])  [unwired: 1 out]
                                n489 = local read "DISPLAY OPTION"() -> (w352:u16)
                                n490 = local read "N°POINTS TO DISPLAY"() -> (w339:i32)
                                n491 = Index Array(array=w335, index=0) -> (element=w347:dbl)
                                n492 = Subtract(x=w335, y=w347) -> (x-y=w348:dbl[])
                                n493 = Divide(x=w348, y=w347) -> (x/y=w346:dbl[])
                                n494 = Equal?(x=w352, y=u16 0) -> (x = y?=w344:bool)
                                n495 = Multiply(x=w346, y=1000000.0 ("f")) -> (x*y=w334:dbl[])
                                n496 = Select(t=w335, s=w344, f=w334) -> (s? t:f=w337:dbl[])
                                n497 = Array Size(array=w337) -> (size(s)=w341:i32)
                                n498 = Subtract(x=w341, y=w339) -> (x-y=w340:i32)
                                n499 = Max & Min(x=0.0, y=w340) -> (max(x,y)=w342:dbl)  [unwired: 1 out]
                                n500 = Array Subset(array=w337, index=w342) -> (w336:dbl[])  [unwired: 1 in]
                              }
                              n501 = local write "TRACK DATA REL"(w330) -> ()
                              n502 = local write "TRACK DATA ABS"(w331) -> ()
                              n503 = local write "LIVE TRACK"(w332) -> ()
                            }
                            frame #11 {
                              n504 = local read "TRACK DATA CLUSTER TBL"() -> (w366:cluster{"CHANNEL":dbl, "KPI 1 TRACK":ext[]}[])
                              n505 = for {
                                tunnel: w366 -> [w379] mode=indexing
                                tunnel: [w370] -> w365 mode=indexing
                                tunnel: [w369] -> w364 mode=indexing
                                n506 = Unbundle By Name(w379) -> ("KPI 1 TRACK"=w368:ext[])
                                n507 = local read "DISPLAY OPTION"() -> (w377:u16)
                                n508 = Delete From Array(array=w368, length=1, index=0) -> (array with subset deleted=w370:ext[])  [unwired: 1 out]
                                n509 = Equal?(x=w377, y=u16 0) -> ()  [unwired: 1 out]
                                n510 = Index Array(array=w370, index=0) -> (element=w372:ext)
                                n511 = Subtract(x=w370, y=w372) -> (x-y=w373:ext[])
                                n512 = Divide(x=w373, y=w372) -> (x/y=w371:ext[])
                                n513 = Multiply(x=w371, y=1000000.0 ("f")) -> (x*y=w369:ext[])
                              }
                              n514 = local write "TRACK DATA ABS NO SMOOTHING"(w365) -> ()
                              n515 = local write "TRACK DATA REL NO SMOOTHING"(w364) -> ()
                            }
                            frame #12 {
                              n516 = local read "TRACK DATA ABS NO SMOOTHING"() -> (w388:dbl[][])
                              n517 = local read "TRACK REPOSITERY"() -> (w401:path)
                              n518 = local read "TRACK REPOSITERY"() -> (w382:path)
                              n519 = local read "TRACK DATA ABS"() -> (w395:dbl[][])
                              n520 = Build Path(base path=w401, name or relative path="ALL CHANNEL ABS Track.txt") -> (appended path=w402:path)
                              n521 = Build Path(base path=w382, name or relative path="ALL CHANNEL ABS Track NS.txt") -> (appended path=w381:path)
                              n522 = call-poly <vilib>:"Write Delimited Spreadsheet.vi"("file path (dialog if empty)"=w402, "format (%.3f)"="%.6f", "2D data"=w395, "transpose? (no:F)"=TRUE) -> ()  [unwired: 10 in, 2 out]
                              n523 = call-poly <vilib>:"Write Delimited Spreadsheet.vi"("file path (dialog if empty)"=w381, "format (%.3f)"="%.6f", "2D data"=w388, "transpose? (no:F)"=TRUE) -> ()  [unwired: 10 in, 2 out]
                              n524 = local read "TRACK DATA REL NO SMOOTHING"() -> (w389:dbl[][])
                              n525 = local read "TRACK REPOSITERY"() -> (w398:path)
                              n526 = local read "TRACK REPOSITERY"() -> (w385:path)
                              n527 = local read "TRACK DATA REL"() -> (w394:dbl[][])
                              n528 = Build Path(base path=w398, name or relative path="ALL CHANNEL REL Track.txt") -> (appended path=w397:path)
                              n529 = Build Path(base path=w385, name or relative path="ALL CHANNEL REL Track NS.txt") -> (appended path=w386:path)
                              n530 = call-poly <vilib>:"Write Delimited Spreadsheet.vi"("file path (dialog if empty)"=w397, "format (%.3f)"="%.6f", "2D data"=w394, "transpose? (no:F)"=TRUE) -> ()  [unwired: 10 in, 2 out]
                              n531 = call-poly <vilib>:"Write Delimited Spreadsheet.vi"("file path (dialog if empty)"=w386, "format (%.3f)"="%.6f", "2D data"=w389, "transpose? (no:F)"=TRUE) -> ()  [unwired: 10 in, 2 out]
                            }
                            frame #13 {
                            }
                          }
                        }
                      }
                    }
                  }
                  frame #2 {
                    n532 = local read "LOOP ACT"() -> (w408:bool)
                    n533 = Select(t="TRACK" ("element"), s=w408, f="WAIT" ("element")) -> (s? t:f=w407:string)
                    n534 = Enqueue Element(queue=w405, element=w407) -> ()  [unwired: 2 in, 3 out]
                  }
                }
              }
              frame "RUN VNA" {
                n535 = local write "STATUS"(w413) -> ()
                n536 = stacked-sequence {
                  tunnel: w411 -> [w437 _]
                  tunnel: w410 -> [w436 _]
                  frame #0 {
                    n537 = local read "RP VNA SETTING"() -> (w432:T1)
                    n538 = local read "SPECTRUM POST PROCESSING PARAMETERS"() -> (w417:cluster{"N° SMOOTHING POINTS":i32})
                    n539 = Unbundle By Name(w417) -> ("N° SMOOTHING POINTS"=w415:i32)
                    n540 = Unbundle By Name(w432) -> ("Sweep size"=w431:u32)
                    n541 = local read "RAW Freq table"() -> (w427:dbl[])
                    n542 = local read "VNA DATA CLUSTER"() -> (w421:T7)
                    n543 = call "VNARP-CASES.vi"("entrée d'erreur (pas d'erreur)"=w436, "Setting"=u32 0, "Énum"=T10."SWEEP START", "ID de connexion"=w437) -> ("sortie d'erreur"=w428:errorcluster, "ID de connexion en sortie"=w433:refnum<k5>)  [unwired: 3 in]
                    n544 = call "VNARP-Read.vi"("ID de connexion"=w433, "entrée d'erreur (pas d'erreur)"=w428, "SIZE"=w431) -> ("MAGNITUDE 1"=w430:sgl[], "PHASE 1"=w429:dbl[])  [unwired: 9 in, 6 out]
                    n545 = call "VNARP-BOXCAR.vi"("Y IN"=w430, "kernel size (pts)"=w415, "Freq table IN"=w427) -> ("Y OUT"=w416:dbl[], "Freq table OUT"=w419:dbl[])  [unwired: 1 in]
                    n546 = call "VNARP-BOXCAR.vi"("Y IN"=w429, "kernel size (pts)"=w415, "Freq table IN"=w427) -> ("Y OUT"=w418:dbl[], "Freq table OUT"=w426:dbl[])  [unwired: 1 in]
                    n547 = Bundle By Name(cluster=w421, "FREQUENCY TABLE"=w419, "MAGNITUDE TABLE"=w416, "PHASE TABLE"=w418) -> (w420:T7)
                    n548 = Build Cluster Array(w419, w416) -> (w424:cluster{dbl, dbl}[])
                    n549 = Build Cluster Array(w426, w418) -> (w425:cluster{dbl, dbl}[])
                    n550 = local write "VNA DATA CLUSTER"(w420) -> ()
                    n551 = Bundle(w424) -> (w423:cluster{cluster{dbl, dbl}[]})  [unwired: 1 in]
                    n552 = Bundle(w425) -> (w422:cluster{cluster{dbl, dbl}[]})  [unwired: 1 in]
                    n553 = Build Array(w423, w422) -> (w414:cluster{cluster{dbl, dbl}[]}[])
                    n554 = local write "MAGNITUDE/PHASE"(w414) -> ()
                    n555 = property on="MAGNITUDE/PHASE" class="XYGraph (strict)"("Val(Sgnl)"=w414) -> ()  [unwired: 2 in, 2 out]
                  }
                  frame #1 {
                    n556 = stacked-sequence {
                      frame #0 {
                        n557 = local write "ACQ Indicator"(TRUE ("ACQ Indicator")) -> ()
                      }
                      frame #1 {
                        n558 = Wait (ms)(milliseconds to wait=u32 100 ("attente (ms)")) -> ()  [unwired: 1 out]
                      }
                      frame #2 {
                        n559 = local write "ACQ Indicator"(FALSE ("ACQ Indicator")) -> ()
                      }
                    }
                  }
                }
                n560 = Wait (ms)(milliseconds to wait=u32 10 ("attente (ms)")) -> ()  [unwired: 1 out]
              }
              frame "CHANNEL CHANGE" {
                n561 = stacked-sequence {
                  frame #0 {
                    n562 = local read "CHANNELS PARAMETERS"() -> (w454:T4)
                    n563 = local read "CHANNEL CHOICE VNA"() -> (w453:T3)
                    n564 = Index Array(array=w454, index=w453) -> (element=w450:T9)
                    n565 = local write "VNA Settings cluster"(w450) -> ()
                    n566 = local read "RP VNA SETTING"() -> (w451:T1)
                    n567 = Unbundle By Name(w450) -> ("START 2"=w444:dbl, "STOP 2"=w449:dbl, "CENTER 2"=w448:dbl, "SPAN 2"=w447:dbl, "PUMP"=w442:dbl, "PROBE"=w443:dbl, "Points N° 2"=w446:i32, "SPACING 2"=w445:dbl)
                    n568 = local write "Points N°"(w446) -> ()
                    n569 = local write "SPACING"(w445) -> ()
                    n570 = local write "CENTER"(w448) -> ()
                    n571 = local write "START"(w444) -> ()
                    n572 = local write "STOP"(w449) -> ()
                    n573 = local write "PROBE"(w443) -> ()
                    n574 = local write "SPAN"(w447) -> ()
                    n575 = local write "PUMP"(w442) -> ()
                    n576 = call "VNARP-VNASETTING CLTR MANAGMENT.vi"("VNA Settings cluster"=w450, "RP VNA SETTING"=w451) -> ("OUTPUT VNA SETTINGS"=w452:T1)  [unwired: 1 in]
                    n577 = local write "RP VNA SETTING"(w452) -> ()
                    n578 = property on="START" class="DigNum (strict)"("Val(Sgnl)"=w444) -> ()  [unwired: 2 in, 2 out]
                  }
                  frame #1 {
                    w463 = u16 0 items=["AOUT0", "AOUT1", "AOUT2", "AOUT3"] ("Pin #")
                    w462 = u16 1 items=["AOUT0", "AOUT1", "AOUT2", "AOUT3"] ("Pin #")
                    n579 = local read "VOA Calibration cluster"() -> (w461:cluster{"PUMP":dbl[], "PROBE":dbl[]})
                    n580 = local read "NETWORK PARAMETERS"() -> (w465:cluster{"RP-IP 1":string, "RP-IP 2":string})
                    n581 = local read "PROBE"() -> (w460:dbl)
                    n582 = Unbundle By Name(w465) -> ("RP-IP 2"=w464:string)
                    n583 = Unbundle By Name(w461) -> ("PUMP"=w455:dbl[], "PROBE"=w459:dbl[])
                    n584 = local read "PUMP"() -> (w456:dbl)
                    n585 = call "RP-VOA CONVERSION P to V.vi"("Calibration points"=w455, "% power"=w456) -> ("DAC Voltage"=w457:dbl)
                    n586 = call "RP-VOA CONVERSION P to V.vi"("Calibration points"=w459, "% power"=w460) -> ("DAC Voltage"=w458:dbl)
                    n587 = call "RP-ANALOG-OUT.vi"("Analog Voltage Value (V)"=w457, "Pin #"=w463, "IP address"=w464) -> ()  [unwired: 1 out]
                    n588 = call "RP-ANALOG-OUT.vi"("Analog Voltage Value (V)"=w458, "Pin #"=w462, "IP address"=w464) -> ()  [unwired: 1 out]
                  }
                  frame #2 {
                    n589 = local read "VNA Settings cluster"() -> (w469:T9)
                    n590 = local read "PROBE"() -> (w467:dbl)
                    n591 = local read "PUMP"() -> (w468:dbl)
                    n592 = Bundle By Name(cluster=w469, "PUMP"=w468, "PROBE"=w467) -> (w466:T9)
                    n593 = local write "VNA Settings cluster"(w466) -> ()
                  }
                  frame #3 {
                    n594 = local read "CHANNELS PARAMETERS"() -> (w475:T4)
                    n595 = local read "CHANNEL CHOICE VNA"() -> (w474:T3)
                    n596 = Index Array(array=w475, index=w474) -> (element=w473:T9)
                    n597 = local read "VNA Settings cluster"() -> (w472:T9)
                    n598 = Unbundle By Name(w473) -> ("CHANNEL TRACK ?"=w471:bool)
                    n599 = Bundle By Name(cluster=w472, "CHANNEL TRACK ?"=w471) -> (w470:T9)
                    n600 = Replace Array Subset(array=w475, new element=w470, index=w474) -> (w476:T4)
                    n601 = local write "CHANNELS PARAMETERS"(w476) -> ()
                  }
                  frame #4 {
                    n602 = local read "CHANNEL CHOICE VNA"() -> (→"CHANNEL CHOSEN":T3)
                  }
                }
              }
              frame "WAIT" {
                n603 = local write "STATUS"(w478) -> ()
              }
              frame "UPDATE" {
                n604 = local write "STATUS"(w483) -> ()
                n605 = stacked-sequence {
                  tunnel: w482 -> [w487 _ _]
                  tunnel: w481 -> [w485 _ _]
                  frame #0 {
                    n606 = local read "RP VNA SETTING"() -> (w486:T1)
                    n607 = call "VNARP-SettingsUpdate.vi"("Error IN"=w485, "RP VNA SETTINGS IN"=w486, "ID de connexion IN"=w487) -> ("Freq table"=w484:dbl[])  [unwired: 2 out]
                    n608 = local write "RAW Freq table"(w484) -> ()
                  }
                  frame #1 {
                    n609 = local read "VNA Settings cluster"() -> (w495:T9)
                    n610 = local read "Points N°"() -> (w489:i32)
                    n611 = local read "SPACING"() -> (w488:dbl)
                    n612 = local read "CENTER"() -> (w491:dbl)
                    n613 = local read "START"() -> (w494:dbl)
                    n614 = local read "SPAN"() -> (w490:dbl)
                    n615 = local read "STOP"() -> (w493:dbl)
                    n616 = Bundle By Name(cluster=w495, "START 2"=w494, "STOP 2"=w493, "CENTER 2"=w491, "SPAN 2"=w490, "Points N° 2"=w489, "SPACING 2"=w488) -> (w492:T9)
                    n617 = local write "VNA Settings cluster"(w492) -> ()
                  }
                  frame #2 {
                    n618 = local read "CHANNELS PARAMETERS"() -> (w501:T4)
                    n619 = local read "CHANNEL CHOICE VNA"() -> (w500:T3)
                    n620 = Index Array(array=w501, index=w500) -> (element=w499:T9)
                    n621 = local read "VNA Settings cluster"() -> (w498:T9)
                    n622 = Unbundle By Name(w499) -> ("CHANNEL TRACK ?"=w497:bool)
                    n623 = Bundle By Name(cluster=w498, "CHANNEL TRACK ?"=w497) -> (w496:T9)
                    n624 = Replace Array Subset(array=w501, new element=w496, index=w500) -> (w502:T4)
                    n625 = local write "CHANNELS PARAMETERS"(w502) -> ()
                  }
                }
              }
              frame "POWER UPDATE" {
                n626 = local write "STATUS"(w503) -> ()
                n627 = stacked-sequence {
                  frame #0 {
                    w513 = u16 0 items=["AOUT0", "AOUT1", "AOUT2", "AOUT3"] ("Pin #")
                    w515 = u16 1 items=["AOUT0", "AOUT1", "AOUT2", "AOUT3"] ("Pin #")
                    n628 = local read "NETWORK PARAMETERS"() -> (w514:cluster{"RP-IP 1":string, "RP-IP 2":string})
                    n629 = local read "VOA Calibration cluster"() -> (w511:cluster{"PUMP":dbl[], "PROBE":dbl[]})
                    n630 = Unbundle By Name(w514) -> ("RP-IP 2"=w512:string)
                    n631 = Unbundle By Name(w511) -> ("PUMP"=w506:dbl[], "PROBE"=w509:dbl[])
                    n632 = local read "PUMP"() -> (w507:dbl)
                    n633 = local read "PROBE"() -> (w510:dbl)
                    n634 = call "RP-VOA CONVERSION P to V.vi"("Calibration points"=w506, "% power"=w507) -> ("DAC Voltage"=w505:dbl)
                    n635 = call "RP-VOA CONVERSION P to V.vi"("Calibration points"=w509, "% power"=w510) -> ("DAC Voltage"=w508:dbl)
                    n636 = call "RP-ANALOG-OUT.vi"("Analog Voltage Value (V)"=w508, "Pin #"=w515, "IP address"=w512) -> ()  [unwired: 1 out]
                    n637 = call "RP-ANALOG-OUT.vi"("Analog Voltage Value (V)"=w505, "Pin #"=w513, "IP address"=w512) -> ()  [unwired: 1 out]
                  }
                  frame #1 {
                    n638 = local read "VNA Settings cluster"() -> (w519:T9)
                    n639 = local read "PROBE"() -> (w517:dbl)
                    n640 = local read "PUMP"() -> (w518:dbl)
                    n641 = Bundle By Name(cluster=w519, "PUMP"=w518, "PROBE"=w517) -> (w516:T9)
                    n642 = local write "VNA Settings cluster"(w516) -> ()
                  }
                  frame #2 {
                    n643 = local read "CHANNELS PARAMETERS"() -> (w525:T4)
                    n644 = local read "CHANNEL CHOICE VNA"() -> (w524:T3)
                    n645 = Index Array(array=w525, index=w524) -> (element=w523:T9)
                    n646 = local read "VNA Settings cluster"() -> (w522:T9)
                    n647 = Unbundle By Name(w523) -> ("CHANNEL TRACK ?"=w521:bool)
                    n648 = Bundle By Name(cluster=w522, "CHANNEL TRACK ?"=w521) -> (w520:T9)
                    n649 = Replace Array Subset(array=w525, new element=w520, index=w524) -> (w526:T4)
                    n650 = local write "CHANNELS PARAMETERS"(w526) -> ()
                  }
                }
              }
              frame "STOP" {
                w528 = FALSE ("TRACK-STOP")
                n651 = local write "STATUS"(w527) -> ()
                n652 = TCP Close Connection(connection ID=w530, error in (no error)=w529) -> ()  [unwired: 1 in, 2 out]
                n653 = local write "TRACK-STOP"(w528) -> ()
                n654 = local write "LOOP ACT"(w528) -> ()
              }
            }
          }
          frame Error {
          }
        }
      }
      n655 = And(x=w62, y=w61) -> (x .and. y?=w60:bool)
      n656 = case shown="True" w60 {
        tunnel: w71 -> [_ w75]
        tunnel: w69 -> [_ w74]
        frame False {
        }
        frame True {
          n657 = Release Queue(queue=w74, error in (no error)=w75) -> ()  [unwired: 1 in, 3 out]
          n658 = property on="MAIN TAB" class="TabCtl (strict)"("Tabs Visible?"=TRUE ("Onglets visibles ?")) -> ()  [unwired: 2 in, 2 out]
        }
      }
    }
  }
